vi "TLB Native Dynamic Events ver 0.13d.vi"() -> ()   [LabVIEW 2018]
uses:
  Labview Training Phase 2/Enum Controls/States for Action Engine.ctl
  TLB Type Definitions/State Type Definitions, for 0.26d versions and later.ctl
  TLB Type Definitions/Intruction Type Definitions.ctl
  TLB Type Definitions/Encoder cluster.ctl
  TLB Type Definitions/PING CLUSTER.ctl
  <vilib>/Studica/Studica Toolkit/NavX/NavX.lvlib
  <vilib>/Studica/Studica Toolkit/Background/DIO Channel.ctl
  Underlying VI's/NavX VI/navX type def.ctl
  <vilib>/myRIO/Instrument Drivers/Utilities/Utilities.lvlib
  <vilib>/Studica/Studica Toolkit/Background/I2C Channel.ctl
  TLB Type Definitions/Vision cluster.ctl
  <vilib>/NI_Real-Time Target Support.lvlib
  TLB Type Definitions/Stepper cluster.ctl
  Experimental VI's/Archived VI's/MOTOR CONTROL NO PID Type Def.ctl
  Underlying VI's/I2C Master VI/I2C MASTER Type Def.ctl
  Underlying VI's/I2C Master VI/I2C_MASTER_WRITE_NEW Type Def.ctl
  Underlying VI's/Webcam FGV Low level ver/State control.ctl
  <vilib>/userdefined/High Color/IMAQdx.ctl
  Underlying VI's/I2C Master VI/Arduino_Interfacing.ctl
  TLB Type Definitions/Yaw Cluster.ctl
  Experimental VI's/Archived VI's/MOTOR CONTROL NO PID AE DATA ENTRY MODE Type def.ctl
  Experimental VI's/Archived VI's/MOTOR CONTROL NO PID AE DIRECTIONS type def.ctl
  <vilib>/Utility/RT CPU Load.ctl
panel:
  out "Task selection":u8
  out "Object Center Coordinates":cluster{"x":sgl, "y":sgl}
  out "Object detection cluster":T1
  in  "Object recognition mode":enum16{"Ball", "Soap", "Gel", "Pipe", "None"}(ring)
  out "NavX Readings":T2
  out "Arduino Data":T3
  out "CPU loads":T4[](array[typedef]) {"ISR (%)" format="%#.2f"; "Idle (%)" format="%#.2f"; "Background (%)" format="%#.2f"; "Normal (%)" format="%#.2f"; "Above Normal (%)" format="%#.2f"; "High (%)" format="%#.2g"; "Timed Structures (%)" format="%#.2g"; "Time Critical (%)" format="%#.2g"; "Total (%)" format="%#.2g"}
  in  "Red LED":bool
  out "Detect?":bool
  out "TASK ENABLE":bool
  out "Rising Edge":bool
  in  "Green LED":bool
  out "Object detected?":bool
  out "I2C Error":errorcluster
  out "State Logic":T5=enum."Startup"
  out "elements":T6[](array[typedef])
  in  "STOP TASK":bool
  in  "OK Button":bool
  in  "STOP":bool
  out "error out":errorcluster
  out "Action Queue Items":i32
  out "State Logic Queue Items":i32
  out "Action Queues items":string[](array[string])=["Hardware reset", "Software reset", ""]
  out "Action State":string
  # "TLB FRAMEWORK STATUS"
  # "System Health Status Update"
  # "Test Programme written by Calvin Loke    Dated: 28 Aug 2019\nTest Programme revised by Dr Alex See   Dated 30 Aug 2019\n\nProgramme version:   TLB Native Dynamic Events ver 0.04b.vi"
  # "VISION"
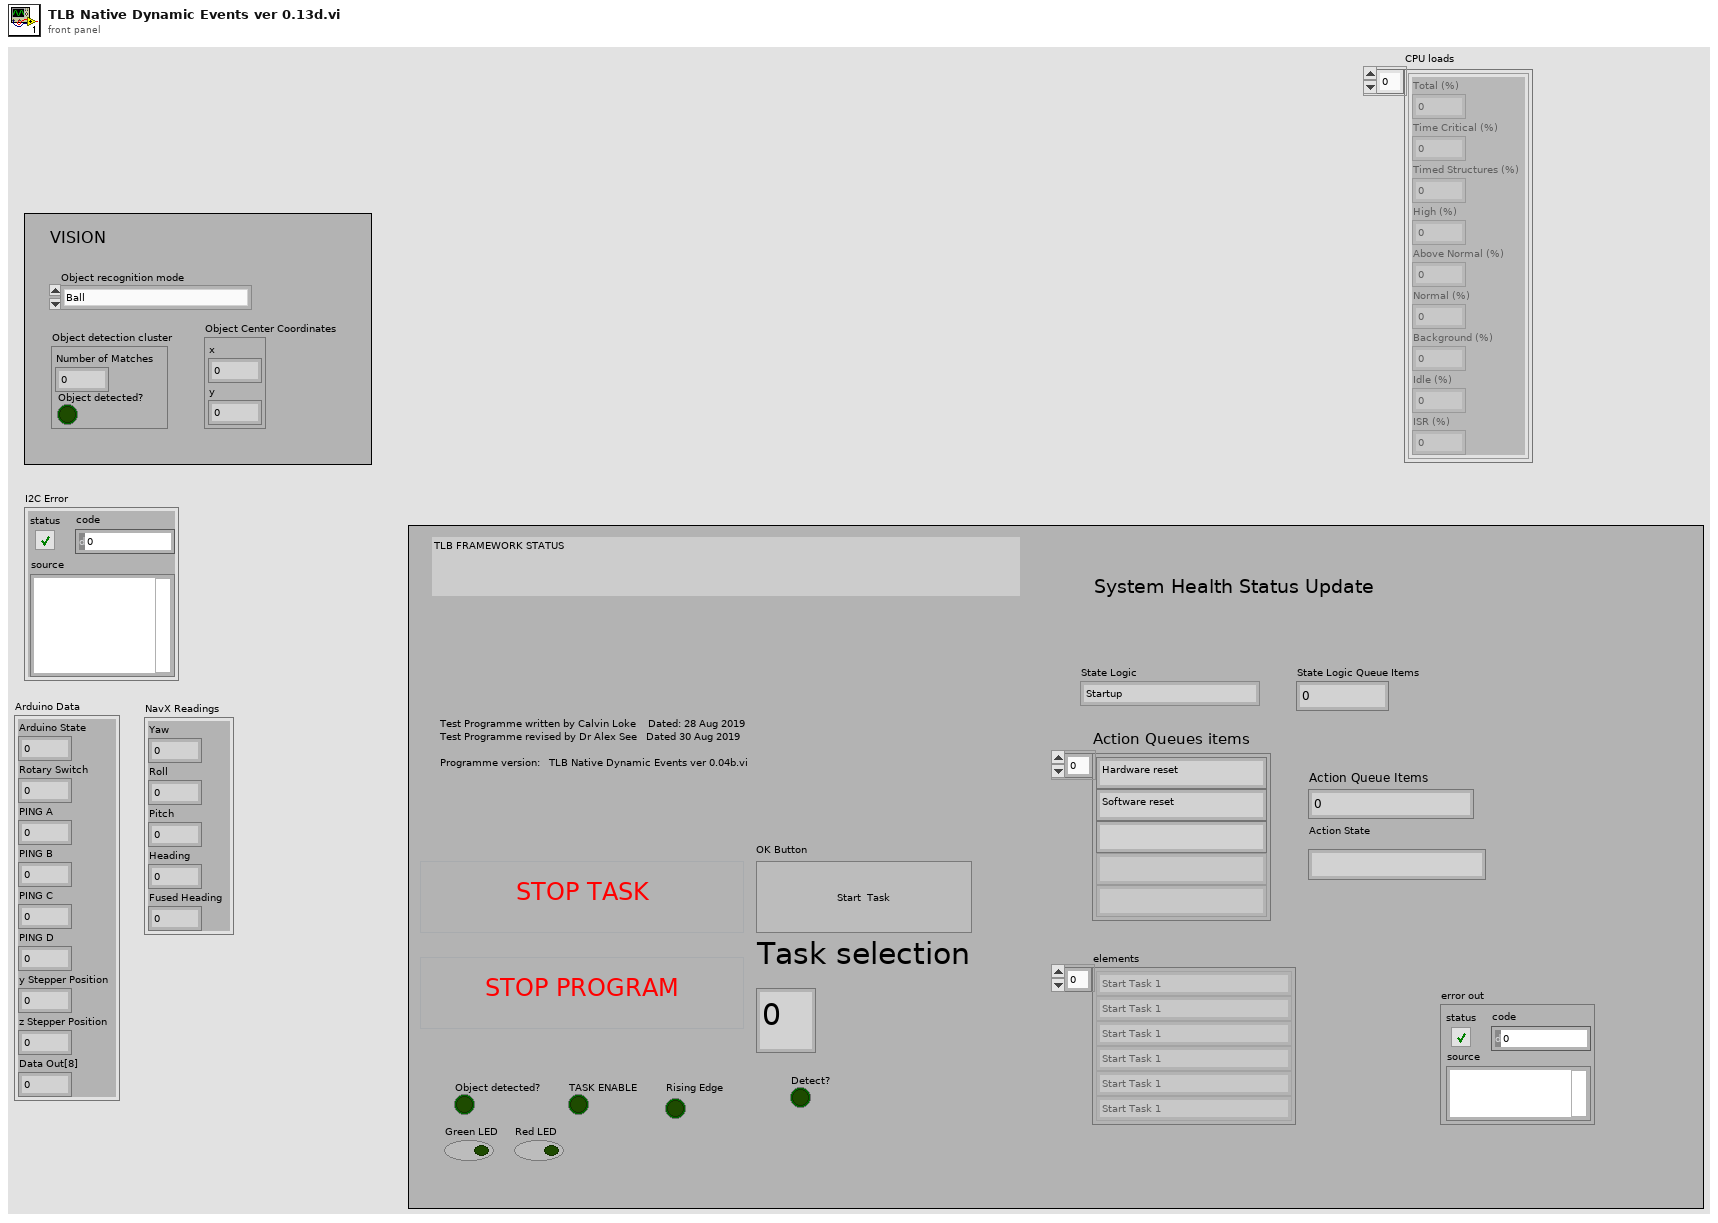
[diagram p1: front panel]
types:
  T1 = cluster{"Number of Matches":i32, "Object detected?":bool}
  T2 = cluster{"Yaw":dbl, "Roll":dbl, "Pitch":dbl, "Heading":dbl, "Fused Heading":dbl}
  T3 = cluster{"Arduino State":u8, "Rotary Switch":u8, "PING A":u8, "PING B":u8, "PING C":u8, "PING D":u8, "y Stepper Position":u8, "z Stepper Position":u8, "Data Out[8]":u8}
  T4 = typedef "NI_Real-Time Target Support.lvlib/RT CPU Load.ctl" = cluster{"Total (%)":dbl, "Time Critical (%)":dbl, "Timed Structures (%)":dbl, "High (%)":dbl, "Above Normal (%)":dbl, "Normal (%)":dbl, "Background (%)":dbl, "Idle (%)":dbl, "ISR (%)":dbl}
  T5 = typedef "State Type Definitions.ctl" = enum16{"None", "Startup", "Move to Angle", "True Stop", "Idle", "Shutdown", "Task 1A", "Task 1B", "Task 2:Raise Arm", "Task 2:Sensor Mode", "Task 2:Reverse Mode", "Task 3", "Task 4_A", "Task 4_B", "Task 4_C", "Task 4_D", "Task 5A", "Task 5B", "Task 5C", "Task 5D", "Task 5E: POSITION ARM", "Task 5F: ARM GRAB HEIGHT", "Task 5G: CLOSE CLAW", "Task 5H: RAISE ARM", "Task 6_A", "Task 6_B", "Task 7", "Task 8A: RAISE ARM", "Task 8B: MOVE TO BOX", "Task 8C: CAM BURST", "Task 8D: PROCESS IMAGE", "Task 8E: ROBOT ADJUST", "Task 8F: CAM BURST 2", "Task 8G: PROCESS IMAGE 2", "Task 8H: ARM ADJUST", "Task 8I: ARM GRAB HEIGHT", "Task 8J: CLOSE CLAW", "Task 8K: RAISE MY SWORD", "Task 9A: Raise Arm", "Task 9B: Rotate to Angle", "Task 9C: Detect Box", "Task 9D: MOVE FORWARD", "Task 9E: MOVE LEFT", "Task 9F: SCAN IMAGE", "Task 9G: PROCESS COLOUR", "Task 9H: MOVE RIGHT", "Task 9I: SCAN IMAGE", "Task 9J: PROCESS COLOUR", "Task 9K: ROTATE 90 CW", "Task 9L: MOVE FORWARD", "Task 9M: MOVE RIGHT", "Task 9N: SCAN IMAGE", "Task 9O: PROCESS COLOUR", "Task 9P: MOVE RIGHT", "Task 9Q: SCAN IMAGE", "Task 9R: PROCESS COLOUR", "Task A1: Raise Arm", "Task A2: Rotate to Angle", "Task A3: Move Forward", "Task A4: Rotate CW 90"}
  T6 = typedef "Intruction Type Definitions.ctl" = enum16{"None", "Start Task 1", "Start Task 2", "Start Task 3", "Start Task 4", "Start Task 5", "Start Task 6", "Start Task 7", "Start Task 8 - BALL", "Start Task 8 - Gel", "Start Task 8 - Pipe", "Start Task 8 - Soap", "Start Task 9", "Start Task A", "Start Task B", "Exit"}
  T7 = typedef "Yaw Cluster.ctl" = cluster{"Yaw":dbl, "Compass":dbl}
  T8 = typedef "Stepper cluster.ctl" = cluster{"y Stepper Position":u8, "z Stepper Position":u8}
  T9 = typedef "DIO Channel.ctl" = enum16{"Not Connected", "A/DIO1", "A/DIO2", "A/DIO3", "A/DIO4", "A/DIO5", "A/DIO6", "A/DIO7", "A/DIO13", "B/DIO1", "B/DIO2", "B/DIO3", "B/DIO4", "B/DIO5", "B/DIO6", "B/DIO7", "B/DIO13", "C/DIO0", "C/DIO1", "C/DIO2", "C/DIO3", "C/DIO4", "C/DIO5", "C/DIO6", "C/DIO7"}
  T10 = typedef "Vision cluster.ctl" = cluster{"Recognized Object":bool, "Object X coordinate":dbl, "Object Y coordinate":dbl}
  T11 = typedef "PING CLUSTER.ctl" = cluster{"PING_A":u8, "PING_B":u8, "PING_C":u8, "PING_D":u8}
  T12 = typedef "Encoder cluster.ctl" = cluster{"xDistance":dbl, "yDistance":dbl, "wDistance":dbl}
  T13 = cluster{"DIO Channel":T9, "FPGA VI Reference Out":refnum<k20>}
  T14 = typedef "navX type def.ctl" = enum16{"Get i2C reference", "Read Values", "Zero Yaw"}
  T15 = typedef "Arduino_Interfacing.ctl" = enum16{"Initialize", "Write to Arduino", "Read From Arduino"}
  T16 = typedef "I2C Channel.ctl" = enum16{"Not Connected", "A", "B"}
  T17 = typedef "States for Action Engine.ctl" = enum16{"Initialize", "Write", "Read"}
  T18 = cluster{"I2C Ref Out":cluster{"I2C Channel":T16, "FPGA VI Reference Out":refnum<k20>}, "Connected":bool, "Slave Address (7-bit)":u8, "Registry":u8[]}
  T19 = typedef "IMAQ Image.ctl" = refnum<image>
  T20 = typedef "State Type Definitions.ctl" = enum16{"None", "Startup", "Move to Angle", "True Stop", "Idle", "Shutdown", "Task 1", "Task 2:Raise Arm", "Task 2:Sensor Mode", "Task 2:Reverse Mode", "Task 3", "Task 4_A", "Task 4_B", "Task 4_C", "Task 4_D", "Task 5A: ARM CAM HEIGHT", "Task 5B: MOVE TO BOX", "Task 5C: CAM BURST", "Task 5D: PROCESS IMAGE", "Task 5E: POSITION ARM", "Task 5F: ARM GRAB HEIGHT", "Task 5G: CLOSE CLAW", "Task 5H: RAISE ARM", "Task 6_A", "Task 6_B", "Task 7", "Task 8A: RAISE ARM", "Task 8B: MOVE TO BOX", "Task 8C: CAM BURST", "Task 8D: PROCESS IMAGE", "Task 8E: ROBOT ADJUST", "Task 8F: CAM BURST 2", "Task 8G: PROCESS IMAGE 2", "Task 8H: ARM ADJUST", "Task 8I: ARM GRAB HEIGHT", "Task 8J: CLOSE CLAW", "Task 8K: RAISE MY SWORD", "Task 9A: Raise Arm", "Task 9B: Rotate to Angle", "Task 9C: Detect Box", "Task 9D: MOVE FORWARD", "Task 9E: MOVE LEFT", "Task 9F: SCAN IMAGE", "Task 9G: PROCESS COLOUR", "Task 9H: MOVE RIGHT", "Task 9I: SCAN IMAGE", "Task 9J: PROCESS COLOUR", "Task 9K: ROTATE 90 CW", "Task 9L: MOVE FORWARD", "Task 9M: MOVE RIGHT", "Task 9N: SCAN IMAGE", "Task 9O: PROCESS COLOUR", "Task 9P: MOVE RIGHT", "Task 9Q: SCAN IMAGE", "Task 9R: PROCESS COLOUR"}
  T21 = typedef "State Type Definitions.ctl" = enum16{"None", "Startup", "Move to Angle", "True Stop", "Idle", "Shutdown", "Task 1", "Task 2", "Task 3", "Task 4_A", "Task 4_B", "Task 4_C", "Task 5", "Task 6_A", "Task 6_B", "Task 7", "Task 8", "Task 9", "Task A", "Task B"}
  T22 = typedef "MOTOR CONTROL NO PID AE DIRECTIONS type def.ctl" = enum16{"y-axis movement", "x-axis movement", "Rotate", "Stop"}
  T23 = typedef "MOTOR CONTROL NO PID AE DATA ENTRY MODE Type def.ctl" = enum16{"Initialize", "Reset Encoders", "Write to motors", "Read from Encoders"}
  T24 = typedef "I2C_MASTER_WRITE_NEW Type Def.ctl" = enum16{"Ultrasonic sensors", "Stepper origin", "zStepper 13.3k", "zStepper 13k", "zStepper 12k", "zStepper 11k", "zStepper 10k", "zStepper 9k", "zStepper 8k", "zStepper 7k", "zStepper 6k", "zStepper 5k", "zStepper 4k", "zStepper 3k", "zStepper 2k", "zStepper 1k", "zStepper 900", "zStepper 800", "zStepper 700", "zStepper 600", "zStepper 500", "zStepper 400", "zStepper 300", "zStepper 200", "zStepper 100", "zStepper 0", "yStepper control", "Open Claw", "Close Claw", "Soft Reset"}
  T25 = typedef "State control.ctl" = enum16{"Initialise", "Start camera", "Continuous Acquisition ", "Stop camera", "Dispose all"}
  T26 = typedef "IMAQdx.ctl" = refnum<k21>
  T27 = cluster{"xSpeed":dbl, "ySpeed":dbl, "wSpeed":dbl, "xDistance":dbl, "yDistance":dbl, "wDistance":dbl}
  T28 = typedef "MOTOR CONTROL NO PID Type Def.ctl" = enum16{"Init", "Front Back", "Left Right", "Rotate", "Stop", "Latch"}
  T29 = typedef "I2C MASTER Type Def.ctl" = enum16{"Last State", "Mode 0", "Mode 1", "Mode 2", "Mode 3", "Mode 4", "Mode 5", "Mode 6", "Mode 7", "Mode 8", "Mode 9", "Mode 10"}
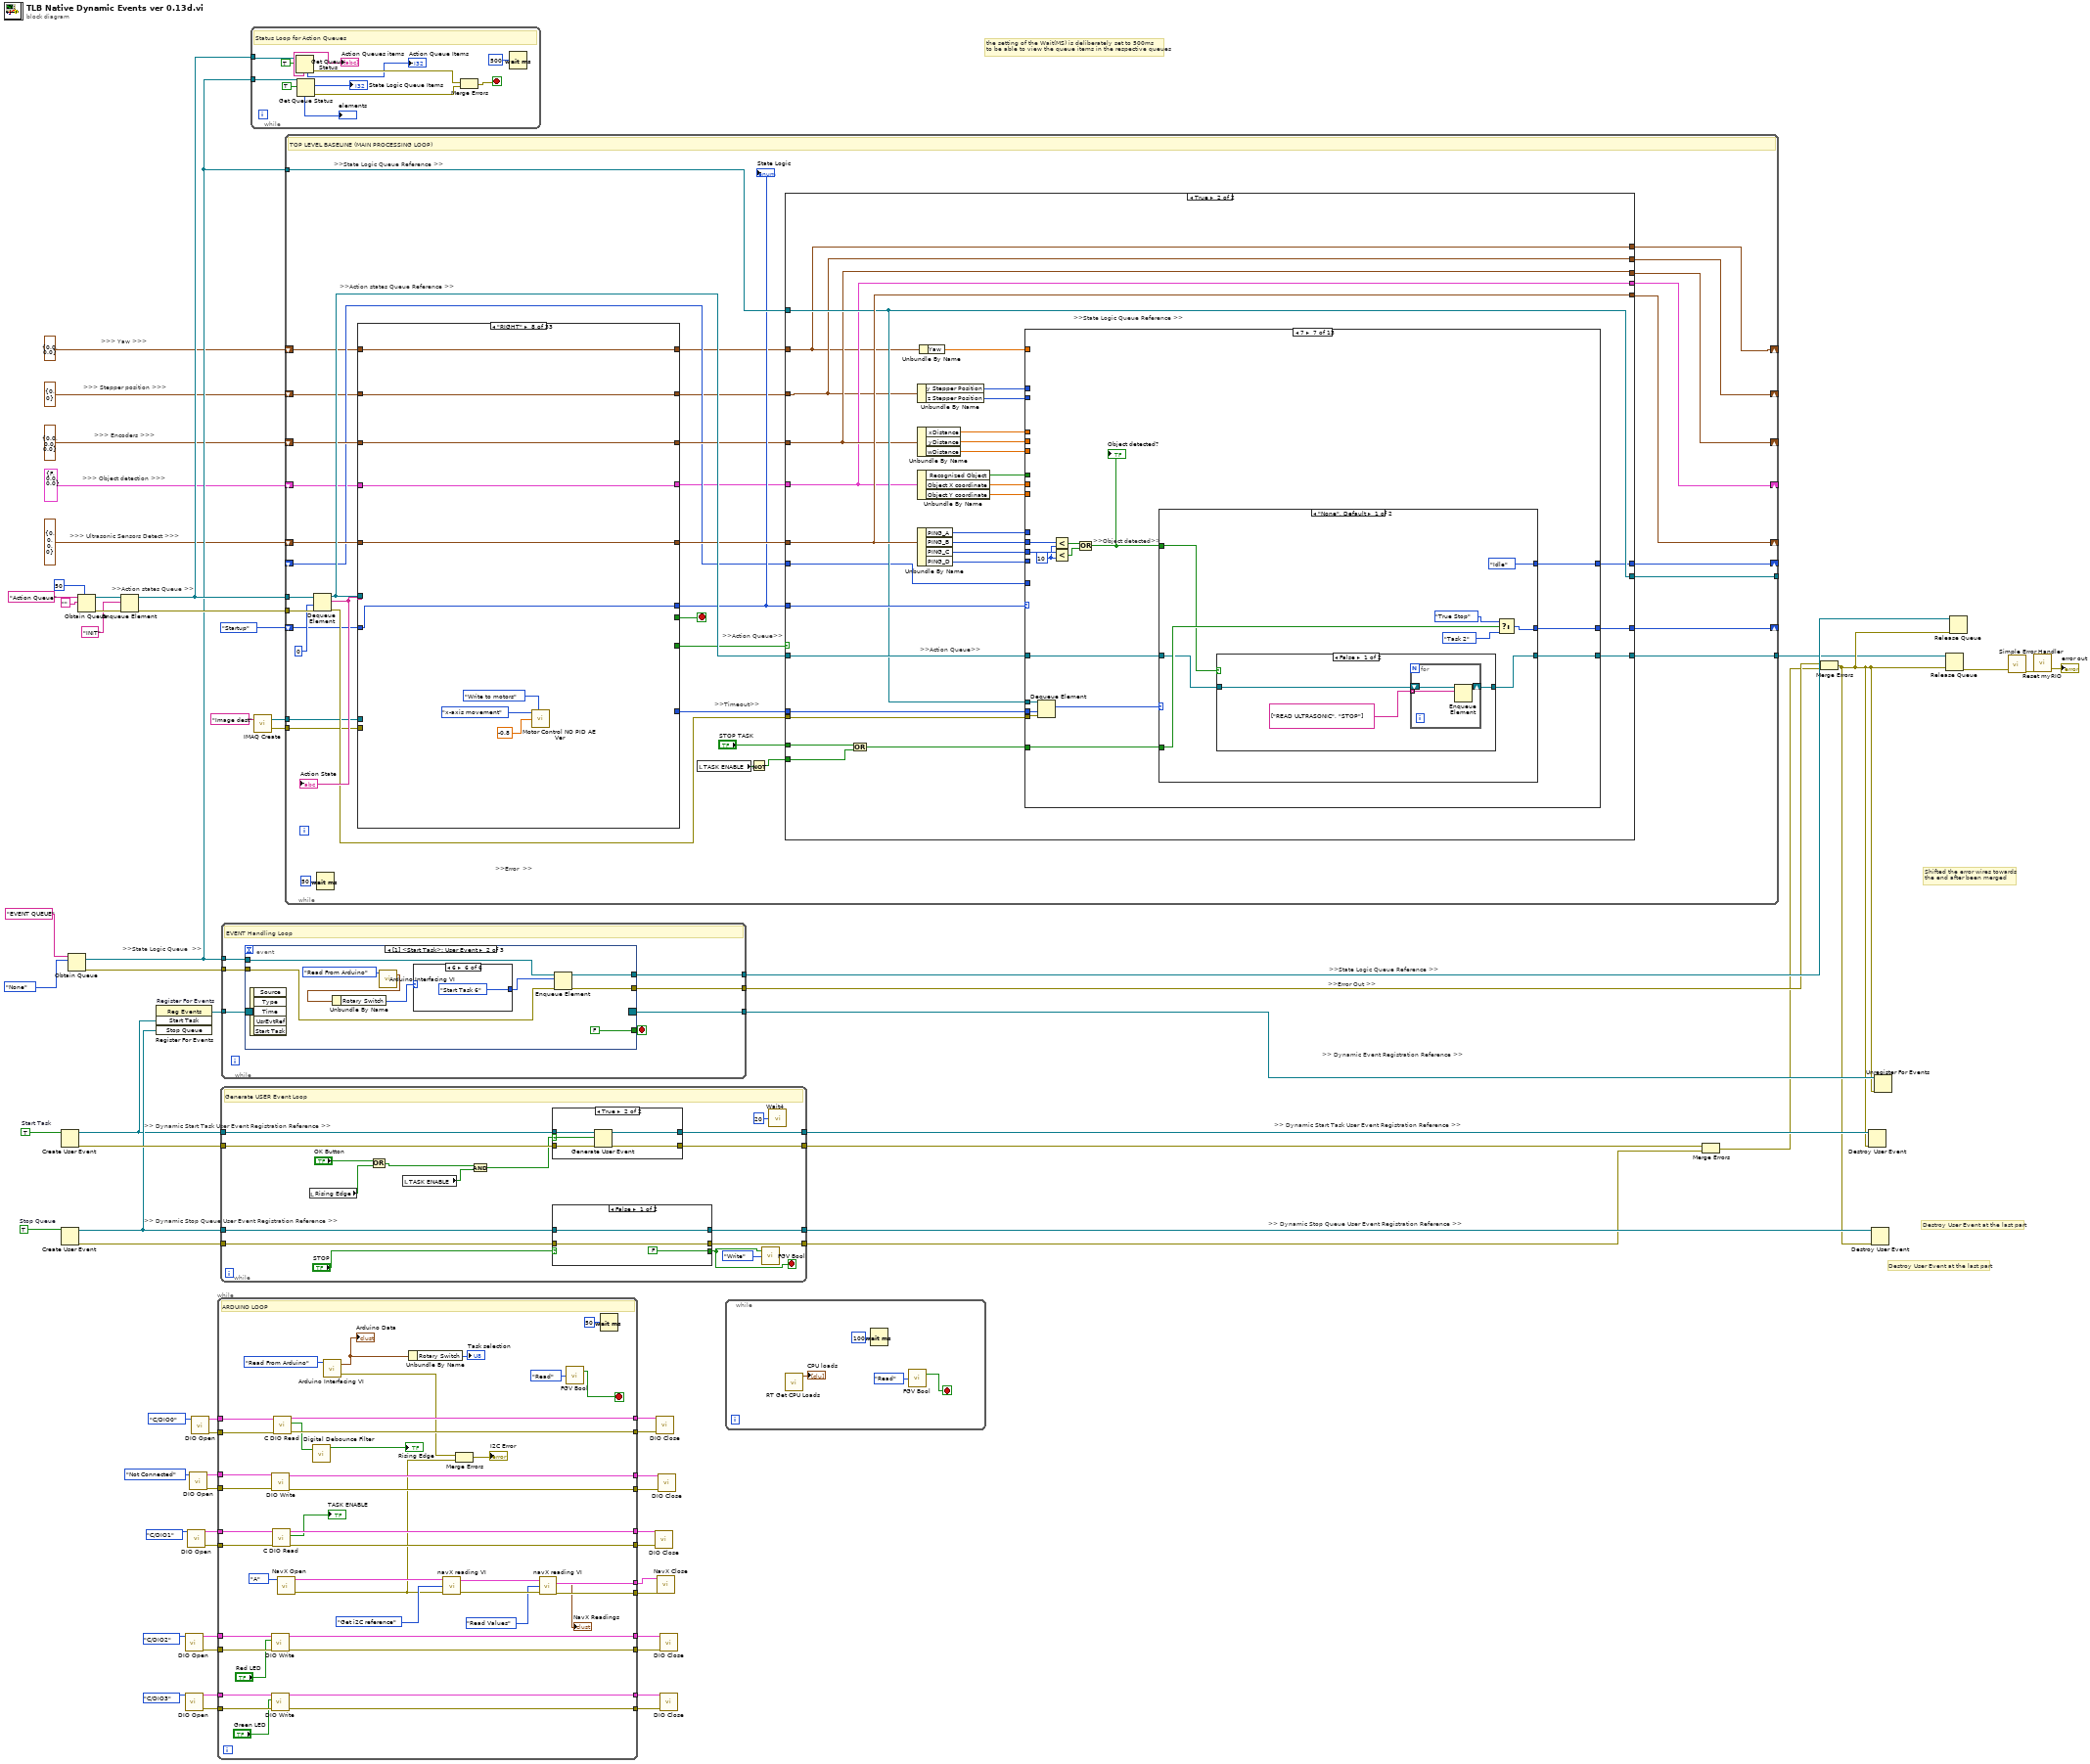
[diagram p0: block diagram]
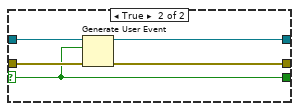
[diagram p2: hidden frame]
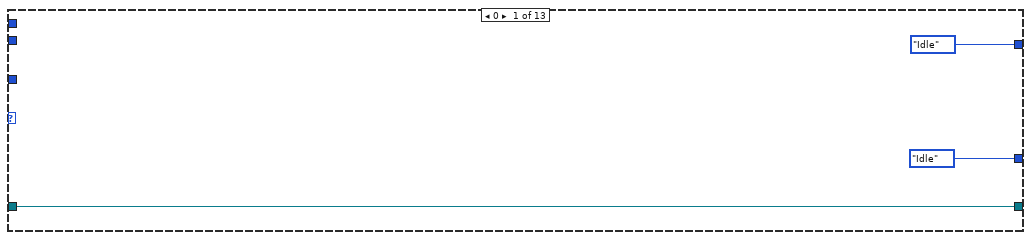
[diagram p5: hidden frame]
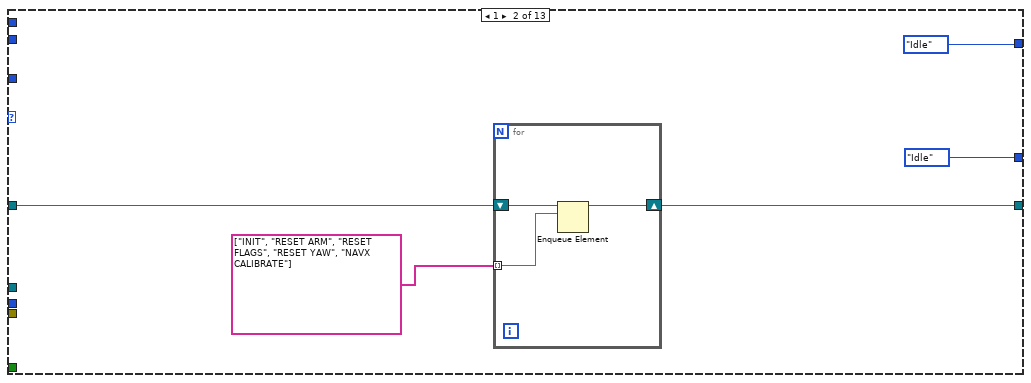
[diagram p6: hidden frame]
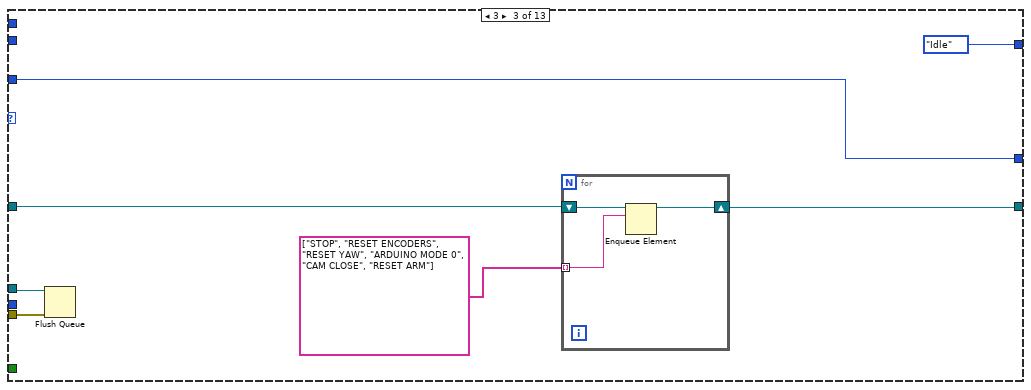
[diagram p7: hidden frame]
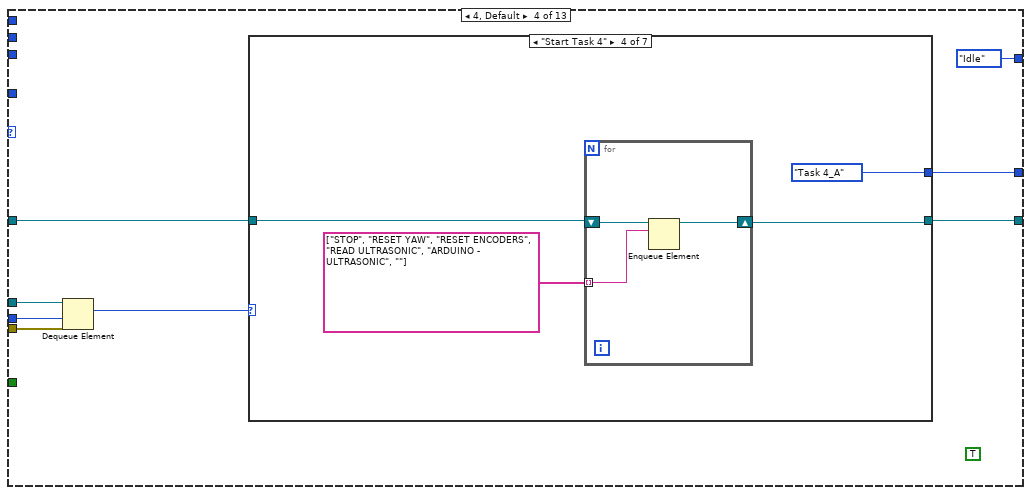
[diagram p8: hidden frame]
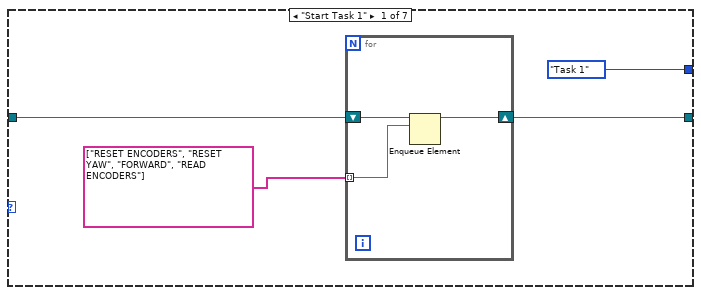
[diagram p9: hidden frame]
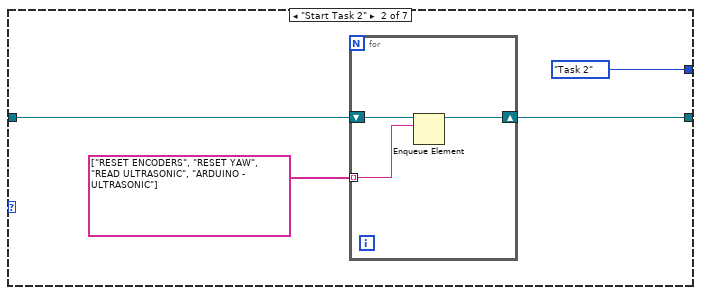
[diagram p10: hidden frame]
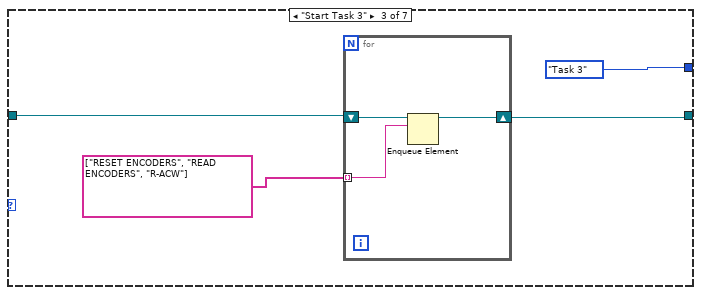
[diagram p11: hidden frame]
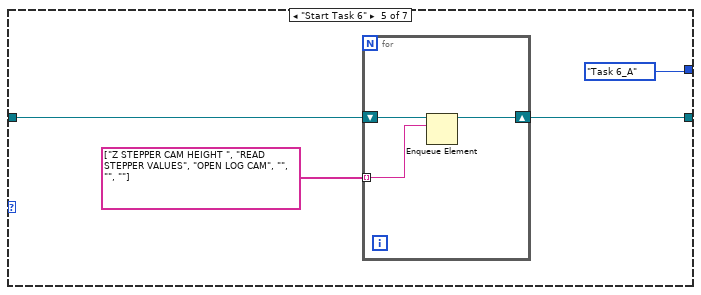
[diagram p12: hidden frame]
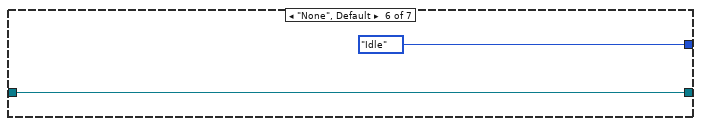
[diagram p13: hidden frame]
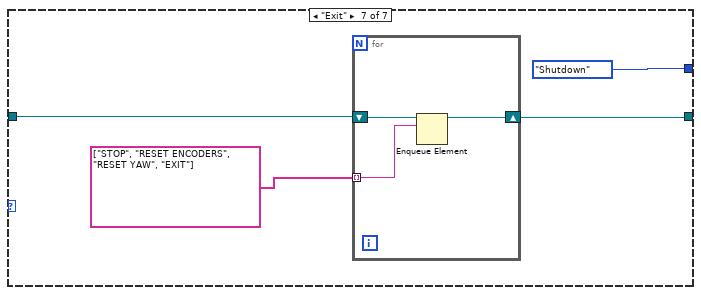
[diagram p14: hidden frame]
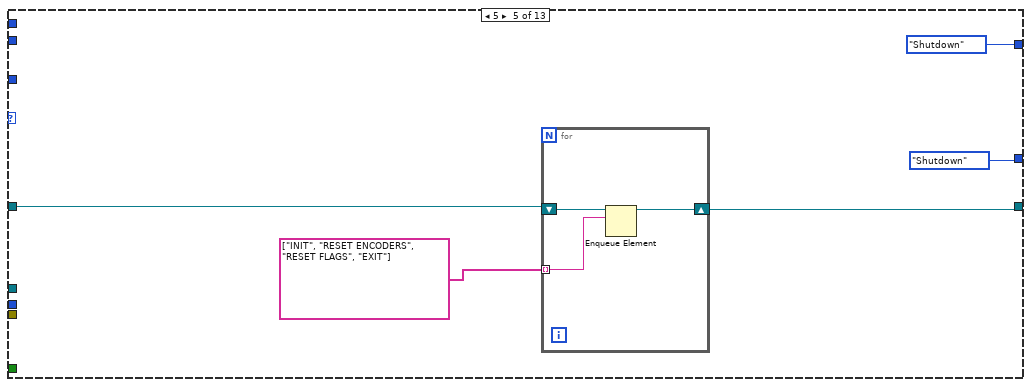
[diagram p15: hidden frame]
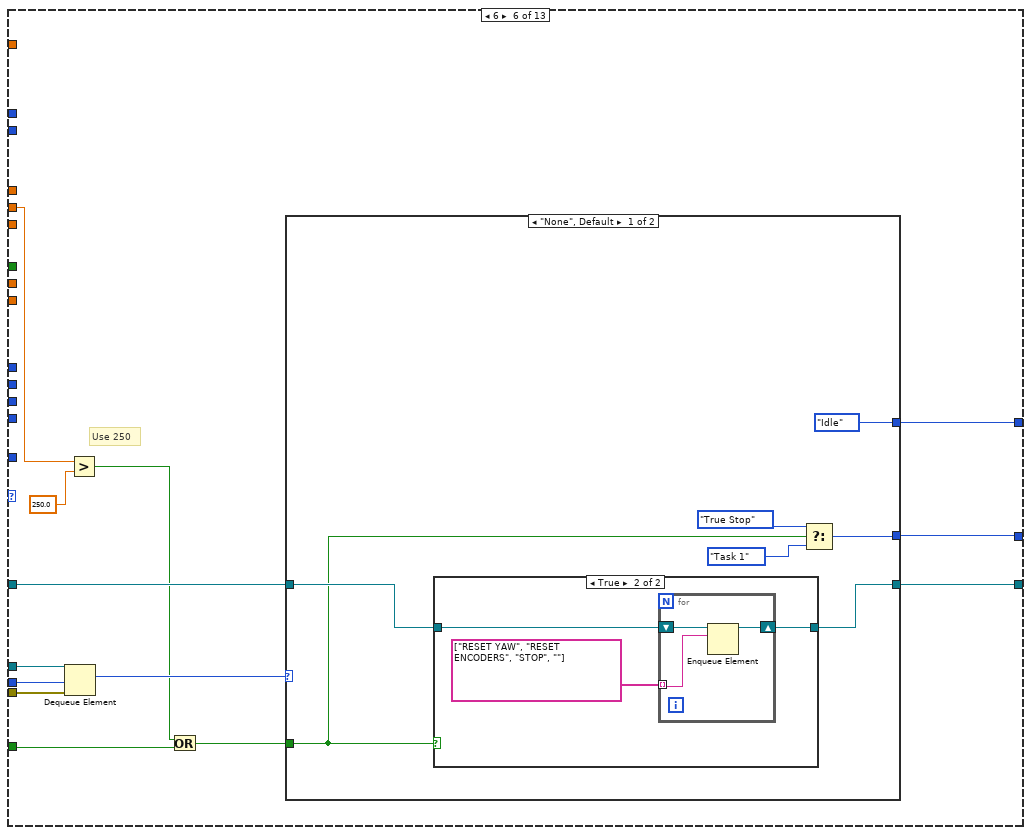
[diagram p16: hidden frame]
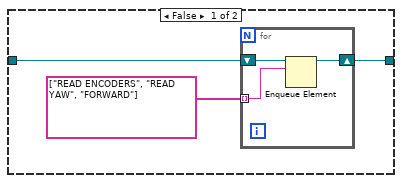
[diagram p17: hidden frame]
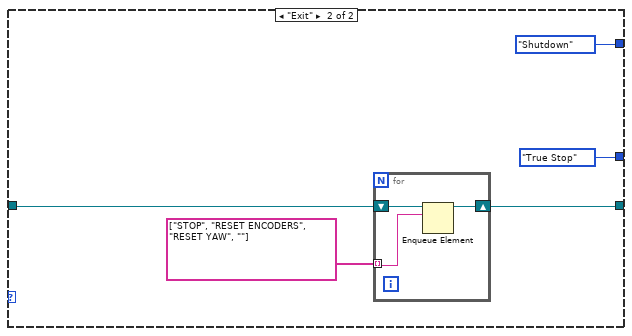
[diagram p18: hidden frame]
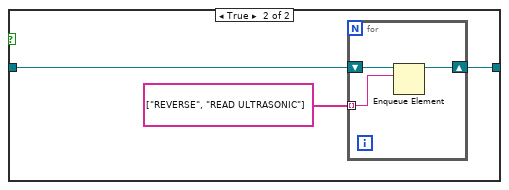
[diagram p19: hidden frame]
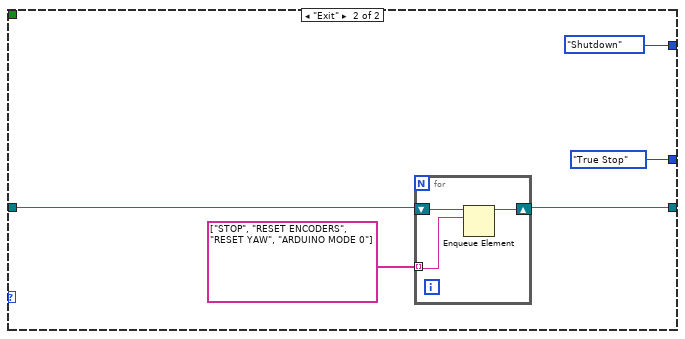
[diagram p20: hidden frame]
diagram:
  w68 = TRUE  # Stop Queue
  w67 = TRUE  # Start Task
  # ">>> Yaw >>>"
  # ">>> Stepper position >>>"
  # ">>> Encoders >>>"
  # ">>> Object detection >>>"
  # ">>> Ultrasonic Sensors Detect >>>"
  # "the setting of the Wait(MS) is deliberately set to 500ms\nto be able to view the queue items in the respective queues"
  # ">>Error Out >>"
  # ">> Dynamic Stop Queue User Event Registration Reference >>"
  # ">> Dynamic Start Task User Event Registration Reference >>"
  # ">> Dynamic Stop Queue User Event Registration Reference >>"
  # ">> Dynamic Start Task User Event Registration Reference >>"
  # ">> Dynamic Event Registration Reference >>"
  # ">>Action states Queue >>"
  # ">>State Logic Queue  >>"
  # ">>State Logic Queue Reference >>"
  # "Destroy User Event at the last part"
  # "Destroy User Event at the last part"
  # "Shifted the error wires towards\nthe end after been merged"
  n1 = Create User Event(user event datatype=w67) -> (user event=w59:refnum<user-event>, error out=w64:errorcluster)  [unwired: 1 in]
  n2 = Create User Event(user event datatype=w68) -> (user event=w60:refnum<user-event>, error out=w63:errorcluster)  [unwired: 1 in]
  n3 = Obtain Queue(name (unnamed)="EVENT QUEUE", element data type=Intruction_Type_Definitions."None" ("Enum")) -> (queue out=w45:refnum<queue>, error out=w51:errorcluster)  [unwired: 3 in, 1 out]
  n4 = Obtain Queue(max queue size (-1, unlimited)=50, name (unnamed)="Action Queue", element data type="") -> (queue out=w54:refnum<queue>, error out=w50:errorcluster)  [unwired: 2 in, 1 out]
  n5 = Enqueue Element(queue=w54, element="INIT", error in (no error)=w50) -> (queue out=w46:refnum<queue>, error out=w49:errorcluster)  [unwired: 1 in, 1 out]
  n6 = register-events "Register For Events"(w59, w60) -> (reference out=w58:refnum<event-registration>)  [unwired: 2 in, 1 out]
  n7 = call <vilib>:"DIO Open.vi"("DIO Channel"=DIO_Channel."C/DIO2") -> ("error out"=w12:errorcluster, "DIO Info Out"=w13:T13)  [unwired: 9 in]
  n8 = call <vilib>:"DIO Open.vi"("DIO Channel"=DIO_Channel."C/DIO3") -> ("error out"=w7:errorcluster, "DIO Info Out"=w8:T13)  [unwired: 9 in]
  n9 = call <vilib>:"DIO Open.vi"("DIO Channel"=DIO_Channel."C/DIO1") -> ("error out"=w23:errorcluster, "DIO Info Out"=w24:T13)  [unwired: 9 in]
  n10 = call <vilib>:"DIO Open.vi"("DIO Channel"=DIO_Channel."Not Connected") -> ("error out"=w28:errorcluster, "DIO Info Out"=w30:T13)  [unwired: 9 in]
  n11 = call <vilib>:"DIO Open.vi"("DIO Channel"=DIO_Channel."C/DIO0") -> ("error out"=w33:errorcluster, "DIO Info Out"=w36:T13)  [unwired: 9 in]
  n12 = while {
    tunnel: w36 -> [w108]
    tunnel: [w107] -> w34
    tunnel: w33 -> [w106]
    tunnel: [w105] -> w32
    tunnel: w30 -> [w101]
    tunnel: [w100] -> w29
    tunnel: w28 -> [w99]
    tunnel: [w98] -> w27
    tunnel: [w97] -> w25
    tunnel: w24 -> [w96]
    tunnel: w23 -> [w95]
    tunnel: [w94] -> w22
    tunnel: w13 -> [w88]
    tunnel: w12 -> [w87]
    tunnel: [w86] -> w11
    tunnel: [w85] -> w10
    tunnel: w8 -> [w83]
    tunnel: w7 -> [w82]
    tunnel: [w81] -> w6
    tunnel: [w80] -> w5
    tunnel: [w74] -> w2
    tunnel: [w73] -> w3
    stop <- w110 stop-if-true
    # "ARDUINO LOOP"
    n13 = call <vilib>:"DIO Write.vi"("error in (no error)"=w87, "Input"="Red LED", "DIO Info In"=w88) -> ("error out"=w85:errorcluster, "DIO Info Out"=w86:T13)  [unwired: 7 in]
    n14 = call <vilib>:"DIO Write.vi"("error in (no error)"=w82, "Input"="Green LED", "DIO Info In"=w83) -> ("error out"=w80:errorcluster, "DIO Info Out"=w81:T13)  [unwired: 7 in]
    n15 = call <vilib>:"DIO Write.vi"("error in (no error)"=w99, "DIO Info In"=w101) -> ("error out"=w98:errorcluster, "DIO Info Out"=w100:T13)  [unwired: 8 in]
    n16 = call <vilib>:"C DIO Read.vi"("error in (no error)"=w95, "DIO Info In in"=w96) -> ("error out"=w94:errorcluster, "IN"=→"TASK ENABLE":bool, "DIO Info In out"=w97:T13)  [unwired: 7 in]
    n17 = call <vilib>:"C DIO Read.vi"("error in (no error)"=w106, "DIO Info In in"=w108) -> ("error out"=w105:errorcluster, "IN"=w103:bool, "DIO Info In out"=w107:T13)  [unwired: 7 in]
    n18 = call <vilib>:"NavX Open.vi"("I2C Channel"=I2C_Channel."A") -> ("error out"=w90:errorcluster, "NavX Info"=w92:T18)  [unwired: 9 in]
    n19 = call "Digital Debounce Filter.vi"("Boolean input"=w103) -> ("Rising Edge"=→"Rising Edge":bool)  [unwired: 1 in, 2 out]
    n20 = call "Arduino Interfacing VI.vi"("AE Mode"=Arduino_Interfacing."Read From Arduino") -> ("error out"=w77:errorcluster, "Arduino Data"=w70:T3)  [unwired: 3 in]
    "Arduino Data" <- w70
    n21 = Unbundle By Name(w70) -> ("Rotary Switch"=→"Task selection":u8)
    n22 = call "navX reading VI.vi"("NavX Info In"=w92, "Mode"=navX_type_def."Get i2C reference", "error in (no error)"=w90) -> ("NavX Info Out"=w76:T18, "Error Out"=w75:errorcluster)  [unwired: 2 out]
    n23 = Merge Errors(w77, w90) -> (→"I2C Error":errorcluster)
    n24 = call "navX reading VI.vi"("NavX Info In"=w76, "Mode"=navX_type_def."Read Values", "error in (no error)"=w75) -> ("NavX Info Out"=w74:T18, "NavX Readings"=→"NavX Readings":T2, "Error Out"=w73:errorcluster)  [unwired: 1 out]
    n25 = call "FGV Bool.vi"("Init/Read/Write State"=States_for_Action_Engine."Read") -> ("Output node"=w110:bool)  [unwired: 2 in, 1 out]
    n26 = Wait (ms)(milliseconds to wait=u32 50) -> ()  [unwired: 1 out]
  }
  n27 = while {
    tunnel: w59 -> [w128]
    tunnel: w60 -> [w127]
    tunnel: [w126] -> w66
    tunnel: [w125] -> w65
    tunnel: w64 -> [w124]
    tunnel: [w123] -> w62
    tunnel: w63 -> [w122]
    tunnel: [w121] -> w61
    stop <- w119 stop-if-true
    # "Generate USER Event Loop"
    n28 = local read "Rising Edge"() -> (w115:bool)
    n29 = Or(x="OK Button", y=w115) -> (x .or. y?=w114:bool)
    n30 = local read "TASK ENABLE"() -> (w113:bool)
    n31 = And(x=w114, y=w113) -> (x .and. y?=w112:bool)
    n32 = case shown="True" w112 {
      selector: w112 -> [_ w139]
      tunnel: w128 -> [w138 w143]
      tunnel: [w138 w142] -> w125
      tunnel: w124 -> [w137 w141]
      tunnel: [w137 w140] -> w123
      frame False {
      }
      frame True {
        n33 = Generate User Event(user event=w143, event data cluster=w139, error in=w141) -> (user event out=w142:refnum<user-event>, error out=w140:errorcluster)  [unwired: 1 in]
      }
    }
    n34 = case shown="False" "STOP" {
      selector: "STOP" -> [_ w132]
      tunnel: w127 -> [w131 w136]
      tunnel: [w131 w135] -> w126
      tunnel: w122 -> [w130 w134]
      tunnel: [w130 w133] -> w121
      tunnel: [FALSE w132] -> w119
      frame False {
      }
      frame True {
        n35 = Generate User Event(user event=w136, event data cluster=w132, error in=w134) -> (user event out=w135:refnum<user-event>, error out=w133:errorcluster)  [unwired: 1 in]
      }
    }
    n36 = call "FGV Bool.vi"("Init/Read/Write State"=States_for_Action_Engine."Write", "Input Node"=w119) -> ()  [unwired: 1 in, 2 out]
    n37 = call "Wait4"("Count(uSec)"=u32 20) -> ()  [unwired: 1 out]
  }
  n38 = while {
    tunnel: w58 -> [w150]
    tunnel: [w149] -> w57
    tunnel: w45 -> [w147]
    tunnel: [w146] -> w56
    tunnel: w51 -> [w145]
    tunnel: [w144] -> w48
    stop <- w148 stop-if-true
    # "EVENT Handling Loop"
    n39 = event shown="[1] <Start Task>: User Event" {
      selector: w150 -> [_ _ _]
      dyn-events: [_ _ _] -> w149
      timeout: _ -> [_ _ _]
      tunnel: [FALSE FALSE w177] -> w148
      tunnel: w147 -> [w155 w164 w175]
      tunnel: [w154 w163 w176] -> w146
      tunnel: w145 -> [w153 w162 w174]
      tunnel: [w152 w161 w173] -> w144
      event Timeout {
        n40 = event-data() -> ()  [unwired: 1 in, 3 out]
        n41 = Enqueue Element(queue=w155, element=Intruction_Type_Definitions."None" ("Enum"), error in (no error)=w153) -> (queue out=w154:refnum<queue>, error out=w152:errorcluster)  [unwired: 1 in, 1 out]
      }
      event User Event {
        n42 = event-data() -> ()  [unwired: 1 in, 5 out]
        n43 = call "Arduino Interfacing VI.vi"("AE Mode"=Arduino_Interfacing."Read From Arduino") -> ("Arduino Data"=w158:T3)  [unwired: 3 in, 1 out]
        n44 = Unbundle By Name(w158) -> ("Rotary Switch"=w157:u8)
        n45 = case shown="6" w157 {
          tunnel: [Intruction_Type_Definitions."None" ("Enum") Intruction_Type_Definitions."Start Task 1" ("Enum") Intruction_Type_Definitions."Start Task 2" ("Enum") Intruction_Type_Definitions."Start Task 3" ("Enum") Intruction_Type_Definitions."Start Task 4" ("Enum") Intruction_Type_Definitions."Start Task 6" ("Enum")] -> w160
          frame 0, Default {
          }
          frame 1 {
          }
          frame 2 {
          }
          frame 3 {
          }
          frame 4 {
          }
          frame 6 {
          }
        }
        n46 = Enqueue Element(queue=w164, element=w160, error in (no error)=w162) -> (queue out=w163:refnum<queue>, error out=w161:errorcluster)  [unwired: 1 in, 1 out]
      }
      event User Event {
        n47 = event-data() -> ("Stop Queue"=w177:bool)  [unwired: 1 in, 4 out]
        n48 = Enqueue Element At Opposite End(queue=w175, element=Intruction_Type_Definitions."Exit" ("Enum"), error in (no error)=w174) -> (queue out=w176:refnum<queue>, error out=w173:errorcluster)  [unwired: 1 in, 1 out]
      }
    }
  }
  n49 = while {
    tunnel: w46 -> [w187]
    tunnel: w45 -> [w184]
    stop <- w181 stop-if-true
    # "Status Loop for Action Queues"
    n50 = Get Queue Status(queue=w187, return elements? (F)=TRUE) -> (error out=w183:errorcluster, # elements in queue=→"Action Queue Items":i32, elements=→"Action Queues items":string[])  [unwired: 1 in, 5 out]
    n51 = Get Queue Status(queue=w184, return elements? (F)=TRUE) -> (# pending remove=→"State Logic Queue Items":i32, error out=w182:errorcluster, elements=→"elements":T6[])  [unwired: 1 in, 5 out]
    n52 = Merge Errors(w183, w182) -> (w181:errorcluster)
    n53 = Wait (ms)(milliseconds to wait=u32 500) -> ()  [unwired: 1 out]
  }
  n54 = call "IMAQ Create"("Image Name"="Image dest") -> ("New Image"=w17:T19, "error out"=w16:errorcluster)  [unwired: 4 in]
  n55 = while {
    tunnel: w45 -> [w215]
    tunnel: w46 -> [w227]
    tunnel: w49 -> [w225]
    tunnel: [w224] -> _
    tunnel: [w223] -> w39
    shift-right: [w216] -> _
    shift-left: T11 {"PING_A"=0, "PING_B"=0, "PING_C"=0, "PING_D"=0} -> [w218]
    shift-right: [w209] -> _
    shift-left: State_Type_Definitions."Startup" ("Enum") -> [w212]
    shift-right: [w205] -> _
    shift-left: T12 {"xDistance"=0.0, "yDistance"=0.0, "wDistance"=0.0} -> [w207]
    shift-right: [w202] -> _
    shift-left: _ -> [w201]
    tunnel: w17 -> [w200]
    tunnel: w16 -> [w199]
    shift-right: [w196] -> _
    shift-left: T10 {"Recognized Object"=FALSE, "Object X coordinate"=0.0, "Object Y coordinate"=0.0} -> [w198]
    shift-right: [w193] -> _
    shift-left: T8 {"y Stepper Position"=0, "z Stepper Position"=0} -> [w195]
    shift-right: [w190] -> _
    shift-left: T7 {"Yaw"=0.0, "Compass"=0.0} -> [w192]
    stop <- w214 stop-if-true
    # ">>Error  >>"
    # ">>Action Queue>>"
    # ">>Timeout>>"
    # ">>Action states Queue Reference >>"
    # ">>State Logic Queue Reference >>"
    # "TOP LEVEL BASELINE (MAIN PROCESSING LOOP)"
    n56 = Dequeue Element(queue=w227, timeout in ms (-1)=0, error in (no error)=w225) -> (queue out=w219:refnum<queue>, element=w226:string, error out=w220:errorcluster)  [unwired: 1 out]
    "Action State" <- w226
    n57 = Wait (ms)(milliseconds to wait=u32 50) -> ()  [unwired: 1 out]
    n58 = case shown="\"RIGHT\"" w226 {
      tunnel: [_ _ _ _ _ _ _ _ _ _ _ _ _ _ _ _ 0 w863 _ _ _ _ _ _ _ _ _ _ _ _ _ _ _] -> w222
      tunnel: w219 -> [_ _ _ _ _ _ _ _ _ _ _ _ _ _ _ _ _ _ _ _ _ _ _ _ _ _ _ _ _ _ _ _ _]
      tunnel: w218 -> [w701 w708 w717 w726 w735 w744 w753 w762 w771 w776 w789 w801 w810 w817 w839 w847 w856 w864 w871 w878 w903 w912 w918 w925 w936 w947 w965 w975 w980 w988 w996 w1004 w1015]
      tunnel: [w701 w708 w717 w726 w735 w744 w753 w762 w771 w776 w789 w802 w810 w817 w840 w847 w856 w864 w871 w878 w902 w912 w918 w925 w936 w947 w965 w975 w980 w988 w996 w1004 w1015] -> w217
      tunnel: [TRUE TRUE _ _ _ _ _ _ _ _ _ _ _ _ _ _ _ _ _ _ _ _ _ _ _ _ _ _ _ _ _ _ _] -> w214
      tunnel: w212 -> [w699 w706 w716 w725 w734 w743 w752 w761 w770 w775 w788 w800 w809 w816 w838 w846 w853 w861 w870 w877 w901 w911 w917 w924 w930 w941 w964 w970 w979 w987 w995 w1003 w1014]
      tunnel: [_ _ _ _ _ _ _ _ _ _ _ _ _ _ _ _ _ TRUE _ _ _ _ _ _ _ _ _ _ _ _ _ _ _] -> w211
      tunnel: [w699 w706 w716 w725 w734 w743 w752 w761 w770 w775 w788 w800 w809 w816 w838 w846 w853 w861 w870 w877 w901 w911 w917 w924 w930 w941 w964 w970 w979 w987 w995 w1003 w1014] -> w210
      tunnel: w207 -> [w698 w705 w715 w724 w733 w742 w751 w760 w769 w777 w787 w799 w811 w818 w837 w848 w852 w860 w872 w879 w891 w910 w920 w926 w937 w948 w966 w976 w982 w990 w998 w1006 w1017]
      tunnel: [w698 w705 w715 w724 w733 w742 w751 w760 w769 w777 w786 w799 w811 w818 w836 w848 w852 w860 w872 w879 w890 w910 w920 w926 w937 w948 w966 w976 w982 w990 w998 w1006 w1017] -> w206
      tunnel: w200 -> [_ _ _ _ _ _ _ _ _ _ _ _ _ _ _ _ _ _ _ _ _ _ _ _ _ _ w959 _ _ _ _ _ _]
      tunnel: w199 -> [_ _ _ _ _ _ _ _ _ _ _ _ _ _ _ _ _ _ _ _ _ _ _ _ _ _ w958 _ _ _ _ _ _]
      tunnel: w198 -> [w697 w704 w714 w723 w732 w741 w749 w759 w768 w774 w785 w798 w803 w815 w828 w845 w851 w859 w869 w876 w896 w908 w919 w923 w929 w940 w957 w969 w981 w989 w997 w1005 w1016]
      tunnel: [w697 w704 w714 w723 w732 w741 w749 w759 w768 w774 w785 w798 w803 w815 w827 w845 w851 w859 w869 w876 w895 w908 w919 w923 w929 w940 w951 w969 w981 w989 w997 w1005 w1016] -> w197
      tunnel: w195 -> [w696 w703 w713 w722 w731 w740 w748 w758 w767 w773 w784 w797 w812 w814 w833 w844 w850 w858 w868 w875 w886 w907 w916 w922 w928 w939 w950 w968 w978 w986 w994 w1002 w1013]
      tunnel: [w696 w703 w713 w722 w731 w740 w748 w758 w767 w773 w784 w797 w812 w814 w832 w844 w850 w858 w868 w875 w885 w907 w916 w922 w928 w939 w950 w968 w978 w986 w994 w1002 w1012] -> w194
      tunnel: w192 -> [w695 w702 w712 w721 w730 w739 w747 w757 w766 w772 w778 w790 w807 w813 w823 w843 w849 w857 w867 w874 w882 w906 w913 w921 w927 w938 w949 w967 w977 w983 w991 w999 w1007]
      tunnel: [w695 w702 w712 w721 w730 w739 w747 w757 w766 w772 w778 w790 w806 w813 w822 w843 w849 w857 w867 w874 w881 w906 w913 w921 w927 w938 w949 w967 w977 w983 w991 w999 w1007] -> w191
      frame "Exit" {
        n59 = call "Imaq Dispose"("All Images? (No)"=TRUE) -> ()  [unwired: 5 in, 1 out]
      }
      frame "----Movement States----" {
      }
      frame "FORWARD" {
        n60 = call "Motor Control NO PID AE Ver.vi"("Direction"=MOTOR_CONTROL_NO_PID_AE_DIRECTIONS_type_def."y-axis movement", "AE Mode"=MOTOR_CONTROL_NO_PID_AE_DATA_ENTRY_MODE_Type_def."Write to motors", "Speed"=0.8) -> ()  [unwired: 2 in, 2 out]
      }
      frame "LEFT" {
        n61 = call "Motor Control NO PID AE Ver.vi"("Direction"=MOTOR_CONTROL_NO_PID_AE_DIRECTIONS_type_def."x-axis movement", "AE Mode"=MOTOR_CONTROL_NO_PID_AE_DATA_ENTRY_MODE_Type_def."Write to motors", "Speed"=-0.8) -> ()  [unwired: 2 in, 2 out]
      }
      frame "R-ACW" {
        n62 = call "Motor Control NO PID AE Ver.vi"("Direction"=MOTOR_CONTROL_NO_PID_AE_DIRECTIONS_type_def."Rotate", "AE Mode"=MOTOR_CONTROL_NO_PID_AE_DATA_ENTRY_MODE_Type_def."Write to motors", "Speed"=0.5) -> ()  [unwired: 2 in, 2 out]
      }
      frame "R-CW" {
        (unwired) -0.2 ("Speed")
        n63 = call "Motor Control NO PID AE Ver.vi"("Direction"=MOTOR_CONTROL_NO_PID_AE_DIRECTIONS_type_def."Rotate", "AE Mode"=MOTOR_CONTROL_NO_PID_AE_DATA_ENTRY_MODE_Type_def."Write to motors", "Speed"=-0.5) -> ()  [unwired: 2 in, 2 out]
      }
      frame "STOP" {
        n64 = Wait (ms)(milliseconds to wait=u32 200) -> ()  [unwired: 1 out]
        n65 = call "Motor Control NO PID AE Ver.vi"("Direction"=MOTOR_CONTROL_NO_PID_AE_DIRECTIONS_type_def."Stop", "AE Mode"=MOTOR_CONTROL_NO_PID_AE_DATA_ENTRY_MODE_Type_def."Write to motors") -> ()  [unwired: 3 in, 2 out]
      }
      frame "RIGHT" {
        n66 = call "Motor Control NO PID AE Ver.vi"("Direction"=MOTOR_CONTROL_NO_PID_AE_DIRECTIONS_type_def."x-axis movement", "AE Mode"=MOTOR_CONTROL_NO_PID_AE_DATA_ENTRY_MODE_Type_def."Write to motors", "Speed"=-0.8) -> ()  [unwired: 2 in, 2 out]
      }
      frame "REVERSE" {
        n67 = call "Motor Control NO PID AE Ver.vi"("Direction"=MOTOR_CONTROL_NO_PID_AE_DIRECTIONS_type_def."y-axis movement", "AE Mode"=MOTOR_CONTROL_NO_PID_AE_DATA_ENTRY_MODE_Type_def."Write to motors", "Speed"=-0.5) -> ()  [unwired: 2 in, 2 out]
      }
      frame "----SENSOR READING---- " {
      }
      frame "READ ENCODERS" {
        # ">>> Current encoder distance >>>"
        # ">>> Ultrasonic Sensors Detect >>>"
        n68 = call "Motor Control NO PID AE Ver.vi"("AE Mode"=MOTOR_CONTROL_NO_PID_AE_DATA_ENTRY_MODE_Type_def."Read from Encoders") -> ("Speed & distance"=w782:T27)  [unwired: 4 in, 1 out]
        n69 = Unbundle By Name(w782) -> ("xDistance"=w781:dbl, "yDistance"=w780:dbl, "wDistance"=w779:dbl)
        n70 = Bundle By Name(cluster=w787, "xDistance"=w781, "yDistance"=w780, "wDistance"=w779) -> (w786:T12)
      }
      frame "READ ULTRASONIC" {
        (unwired) navX_type_def."Read Values" ("Mode")
        (unwired) MOTOR_CONTROL_NO_PID_Type_Def."Latch" ("Direction")
        # ">>> Ultrasonic Sensors Detect >>>"
        # ">>> Object detection >>>"
        # ">>> Encoders >>>"
        # ">>> Stepper position >>>"
        # ">>> Yaw >>>"
        n71 = call "Arduino Interfacing VI.vi"("AE Mode"=Arduino_Interfacing."Read From Arduino") -> ("Arduino Data"=w795:T3)  [unwired: 3 in, 1 out]
        n72 = Unbundle By Name(w795) -> ("PING A"=w794:u8, "PING B"=w793:u8, "PING C"=w792:u8, "PING D"=w791:u8)
        n73 = Bundle By Name(cluster=w801, "PING_A"=w794, "PING_B"=w793, "PING_C"=w792, "PING_D"=w791) -> (w802:T11)
      }
      frame " READ YAW" {
        # ">>> Yaw >>>"
        # ">>> Ultrasonic Sensors Detect >>>"
        # ">>> Object detection >>>"
        # ">>> Encoders >>>"
        # ">>> Stepper position >>>"
        n74 = call "navX reading VI.vi"("Mode"=navX_type_def."Read Values") -> ("NavX Readings"=w805:T2)  [unwired: 2 in, 3 out]
        n75 = Unbundle By Name(w805) -> ("Yaw"=w804:dbl)
        n76 = Bundle By Name(cluster=w807, "Yaw"=w804) -> (w806:T7)
      }
      frame "----SYSTEM MODES----" {
        (unwired) I2C_MASTER_Type_Def."Last State" ("Arduino Mode")
        # ">>> Object detection >>>"
        # ">>> Yaw >>>"
        # ">>> Ultrasonic Sensors Detect >>>"
        # ">>> Encoders >>>"
        # ">>> Stepper position >>>"
      }
      frame "INIT" {
        w834 = u8 0
        w835 = 0.0
        # ">>> Object detection >>>"
        # ">>> Yaw >>>"
        # ">>> Ultrasonic Sensors Detect >>>"
        # ">>> Encoders >>>"
        # ">>> Stepper position >>>"
        # ">>State Logic  >>"
        n77 = call "Arduino Interfacing VI.vi"("AE Mode"=Arduino_Interfacing."Initialize") -> ()  [unwired: 3 in, 2 out]
        n78 = call "FGV Bool.vi"("Init/Read/Write State"=States_for_Action_Engine."Initialize") -> ()  [unwired: 2 in, 2 out]
        n79 = call "Motor Control NO PID AE Ver.vi"("AE Mode"=MOTOR_CONTROL_NO_PID_AE_DATA_ENTRY_MODE_Type_def."Initialize") -> ()  [unwired: 4 in, 2 out]
        n80 = Bundle By Name(cluster=w828, "Recognized Object"=FALSE, "Object X coordinate"=0.0, "Object Y coordinate"=0.0) -> (w827:T10)
        n81 = Bundle By Name(cluster=w833, "y Stepper Position"=u8 0, "z Stepper Position"=u8 0) -> (w832:T8)
        n82 = Bundle By Name(cluster=w837, "xDistance"=w835, "yDistance"=w835, "wDistance"=w835) -> (w836:T12)
        n83 = Bundle By Name(cluster=w839, "PING_A"=w834, "PING_B"=w834, "PING_C"=w834, "PING_D"=w834) -> (w840:T11)
        n84 = Bundle By Name(cluster=w823, "Yaw"=0.0) -> (w822:T7)
      }
      frame "ARDUINO - ULTRASONIC" {
        # ">>> Object detection >>>"
        # ">>> Yaw >>>"
        # ">>> Ultrasonic Sensors Detect >>>"
        # ">>> Encoders >>>"
        # ">>> Stepper position >>>"
        # ">>State Logic  >>"
        n85 = call "Arduino Interfacing VI.vi"("Data to Write"=I2C_MASTER_WRITE_NEW_Type_Def."Ultrasonic sensors", "AE Mode"=Arduino_Interfacing."Write to Arduino") -> ()  [unwired: 2 in, 2 out]
      }
      frame "NAVX CALIBRATE" {
        # ">>> Object detection >>>"
        # ">>> Yaw >>>"
        # ">>> Ultrasonic Sensors Detect >>>"
        # ">>> Encoders >>>"
        # ">>> Stepper position >>>"
        # ">>State Logic  >>"
        # "Adds a 15 second delay to the startup process \nfor the NavX to calibrate"
        n86 = Wait (ms)(milliseconds to wait=u32 5000) -> ()  [unwired: 1 out]
      }
      frame "NO ACTION", Default {
        (unwired) u8 0 ("y Stepper value")
        (unwired) TRUE ("Latch")
        (unwired) navX_type_def."Read Values" ("Mode")
        (unwired) MOTOR_CONTROL_NO_PID_Type_Def."Latch" ("Direction")
        # ">>> Object detection >>>"
        # ">>> Yaw >>>"
        # ">>> Ultrasonic Sensors Detect >>>"
        # ">>> Encoders >>>"
        # ">>> Stepper position >>>"
        # ">>State Logic  >>"
        n87 = case shown="4" w861 {
          tunnel: [0 100] -> w863
          frame 1, Default {
          }
          frame 4 {
          }
        }
      }
      frame "----RESET CASES----" {
        (unwired) I2C_MASTER_Type_Def."Last State" ("Arduino Mode")
        # ">>> Object detection >>>"
        # ">>> Yaw >>>"
        # ">>> Ultrasonic Sensors Detect >>>"
        # ">>> Encoders >>>"
        # ">>> Stepper position >>>"
        # ">>State Logic  >>"
      }
      frame "RESET ENCODERS" {
        # ">>> Object detection >>>"
        # ">>> Yaw >>>"
        # ">>> Ultrasonic Sensors Detect >>>"
        # ">>> Encoders >>>"
        # ">>> Stepper position >>>"
        # ">>State Logic  >>"
        n88 = call "Motor Control NO PID AE Ver.vi"("AE Mode"=MOTOR_CONTROL_NO_PID_AE_DATA_ENTRY_MODE_Type_def."Reset Encoders") -> ()  [unwired: 4 in, 2 out]
      }
      frame "RESET FLAGS" {
        (unwired) I2C_MASTER_Type_Def."Last State" ("Arduino Mode")
        # "Resets any software variables\nand/or non-critical states"
        n89 = Wait (ms)(milliseconds to wait=u32 20) -> ()  [unwired: 1 out]
        n90 = Bundle By Name(cluster=w896, "Recognized Object"=FALSE, "Object X coordinate"=0.0, "Object Y coordinate"=0.0) -> (w895:T10)
        n91 = Bundle By Name(cluster=w886, "y Stepper Position"=u8 0, "z Stepper Position"=u8 0) -> (w885:T8)
        n92 = Bundle By Name(cluster=w891, "xDistance"=0.0, "yDistance"=0.0, "wDistance"=0.0) -> (w890:T12)
        n93 = Bundle By Name(cluster=w903, "PING_A"=u8 0, "PING_B"=u8 0, "PING_C"=u8 0, "PING_D"=u8 0) -> (w902:T11)
        n94 = Bundle By Name(cluster=w882, "Yaw"=0.0) -> (w881:T7)
      }
      frame "RESET YAW" {
        n95 = Wait (ms)(milliseconds to wait=u32 100) -> ()  [unwired: 1 out]
        n96 = call "navX reading VI.vi"("Mode"=navX_type_def."Zero Yaw") -> ()  [unwired: 2 in, 4 out]
      }
      frame "RESET ARM" {
        n97 = call "Arduino Interfacing VI.vi"("Data to Write"=I2C_MASTER_WRITE_NEW_Type_Def."Soft Reset", "AE Mode"=Arduino_Interfacing."Write to Arduino") -> ()  [unwired: 2 in, 2 out]
      }
      frame "--------CAM STATES-------" {
      }
      frame "OPEN LOG CAM" {
        n98 = call "Low-Level Grab.vi"("States"=State_control."Initialise", "Session In"=T26 "cam0") -> ("error out"=w932:errorcluster, "Session Out"=w933:T26)  [unwired: 7 in, 1 out]
        n99 = call "Low-Level Grab.vi"("error in (no error)"=w932, "States"=State_control."Start camera", "Session In"=w933) -> ()  [unwired: 6 in, 3 out]
      }
      frame "OPEN LIFE CAM" {
        (unwired) MOTOR_CONTROL_NO_PID_Type_Def."Latch" ("Direction")
        (unwired) navX_type_def."Read Values" ("Mode")
        n100 = call "Low-Level Grab.vi"("States"=State_control."Initialise", "Session In"=T26 "cam1") -> ("error out"=w943:errorcluster, "Session Out"=w944:T26)  [unwired: 7 in, 1 out]
        n101 = call "Low-Level Grab.vi"("error in (no error)"=w943, "States"=State_control."Start camera", "Session In"=w944) -> ()  [unwired: 6 in, 3 out]
      }
      frame "CAM ACQ" {
        # ">>> Yaw >>>"
        # ">>> Stepper position >>>"
        # ">>> Encoders >>>"
        # ">>> Object detection >>>"
        # ">>> Ultrasonic Sensors Detect >>>"
        # "Object detection"
        n102 = call "Low-Level Grab.vi"("error in (no error)"=w958, "States"=State_control."Continuous Acquisition ") -> ("error out"=w961:errorcluster, "Image Out"=w962:T19)  [unwired: 7 in, 1 out]
        n103 = call "Object Detection SubVI.vi"("Error In"=w961, "Mode"="Object recognition mode", "Image Dest"=w959, "Image in"=w962) -> ("Object Center Coordinates"=w956:cluster{"x":sgl, "y":sgl}, "Object detection cluster"=w953:T1)  [unwired: 2 out]
        "Object detection cluster" <- w953
        "Object Center Coordinates" <- w956
        n104 = Unbundle By Name(w953) -> ("Object detected?"=w952:bool)
        n105 = Unbundle By Name(w956) -> ("x"=w955:sgl, "y"=w954:sgl)
        n106 = Bundle By Name(cluster=w957, "Recognized Object"=w952, "Object X coordinate"=w955, "Object Y coordinate"=w954) -> (w951:T10)
      }
      frame "CAM CLOSE" {
        (unwired) MOTOR_CONTROL_NO_PID_Type_Def."Latch" ("Direction")
        (unwired) navX_type_def."Read Values" ("Mode")
        n107 = call "Low-Level Grab.vi"("States"=State_control."Stop camera") -> ("error out"=w972:errorcluster, "Session Out"=w973:T26)  [unwired: 8 in, 1 out]
        n108 = call "Low-Level Grab.vi"("error in (no error)"=w972, "States"=State_control."Dispose all", "Session In"=w973) -> ()  [unwired: 6 in, 3 out]
      }
      frame "-----ARM ACTIONS-----" {
      }
      frame "CLOSE CLAW" {
        n109 = call "Arduino Interfacing VI.vi"("Data to Write"=I2C_MASTER_WRITE_NEW_Type_Def."Close Claw", "AE Mode"=Arduino_Interfacing."Write to Arduino") -> ()  [unwired: 2 in, 2 out]
      }
      frame "OPEN CLAW" {
        n110 = call "Arduino Interfacing VI.vi"("Data to Write"=I2C_MASTER_WRITE_NEW_Type_Def."Open Claw", "AE Mode"=Arduino_Interfacing."Write to Arduino") -> ()  [unwired: 2 in, 2 out]
      }
      frame "Z STEPPER CAM HEIGHT " {
        n111 = call "Arduino Interfacing VI.vi"("Data to Write"=I2C_MASTER_WRITE_NEW_Type_Def."zStepper 10k", "AE Mode"=Arduino_Interfacing."Write to Arduino") -> ()  [unwired: 2 in, 2 out]
      }
      frame "READ STEPPER VALUES" {
        n112 = call "Arduino Interfacing VI.vi"("AE Mode"=Arduino_Interfacing."Read From Arduino") -> ("Arduino Data"=w1010:T3)  [unwired: 3 in, 1 out]
        n113 = Unbundle By Name(w1010) -> ("y Stepper Position"=w1009:u8, "z Stepper Position"=w1008:u8)
        n114 = Bundle By Name(cluster=w1013, "y Stepper Position"=w1009, "z Stepper Position"=w1008) -> (w1012:T8)
      }
    }
    "State Logic" <- w210
    n115 = local read "TASK ENABLE"() -> (w204:bool)
    n116 = Not(x=w204) -> (.not. x?=w203:bool)
    n117 = case shown="True" w211 {
      tunnel: w215 -> [w236 w261]
      tunnel: w219 -> [w232 w263]
      tunnel: [w236 w261] -> w224
      tunnel: [w232 w264] -> w223
      tunnel: w220 -> [_ w259]
      tunnel: w222 -> [_ w260]
      tunnel: w217 -> [w235 w266]
      tunnel: [w235 w266] -> w216
      tunnel: "STOP TASK" -> [_ w249]
      tunnel: w210 -> [w234 w265]
      tunnel: [w234 w262] -> w209
      tunnel: w206 -> [w233 w255]
      tunnel: [w233 w255] -> w205
      tunnel: w203 -> [_ w250]
      tunnel: [w231 w247] -> w202
      tunnel: w201 -> [w231 w246]
      tunnel: w197 -> [w230 w243]
      tunnel: [w230 w243] -> w196
      tunnel: w194 -> [w229 w239]
      tunnel: [w229 w239] -> w193
      tunnel: w191 -> [w228 w237]
      tunnel: [w228 w237] -> w190
      frame False {
      }
      frame True {
        # ">>Action Queue>>"
        # ">>State Logic Queue Reference >>"
        n118 = Or(x=w249, y=w250) -> (x .or. y?=w248:bool)
        n119 = Unbundle By Name(w239) -> ("y Stepper Position"=w241:u8, "z Stepper Position"=w240:u8)
        n120 = Unbundle By Name(w255) -> ("xDistance"=w252:dbl, "yDistance"=w253:dbl, "wDistance"=w254:dbl)
        n121 = Unbundle By Name(w243) -> ("Recognized Object"=w242:bool, "Object X coordinate"=w245:dbl, "Object Y coordinate"=w244:dbl)
        n122 = Unbundle By Name(w266) -> ("PING_A"=w258:u8, "PING_B"=w257:u8, "PING_C"=w256:u8, "PING_D"=w251:u8)
        n123 = Unbundle By Name(w237) -> ("Yaw"=w238:dbl)
        n124 = case shown="7" w265 {
          tunnel: [w268 w271 w282 w289 w341 w353 w389 w435 w479 w536 w573 w625 w666] -> w264
          tunnel: w263 -> [w268 w274 w283 w292 w343 w354 w390 w436 w485 w529 w577 w620 w657]
          tunnel: [State_Type_Definitions."Idle" ("Enum") State_Type_Definitions."Idle" ("Enum") w278 w291 State_Type_Definitions."Shutdown" ("Enum") w355 w392 w434 w480 w535 w574 w626 w658] -> w262
          tunnel: w261 -> [_ _ w281 w295 _ w360 w402 w443 w484 w533 w578 w623 w665]
          tunnel: w260 -> [_ _ _ w294 _ w359 w401 w442 w483 w532 w570 w622 w663]
          tunnel: w259 -> [_ _ w280 w290 _ w358 w400 w441 w482 w531 w569 w621 w664]
          tunnel: w248 -> [_ _ _ _ _ w352 w391 w438 w478 w534 w575 w624 w661]
          tunnel: w258 -> [_ _ _ _ _ _ _ _ _ _ _ _ _]
          tunnel: w257 -> [_ _ _ _ _ _ w398 _ w476 w524 w580 _ _]
          tunnel: w256 -> [_ _ _ _ _ _ w397 _ w477 w525 w579 _ _]
          tunnel: w254 -> [_ _ _ _ _ _ _ w440 _ _ _ _ _]
          tunnel: w253 -> [_ _ _ _ _ w351 _ _ _ _ _ _ _]
          tunnel: w252 -> [_ _ _ _ _ _ _ _ _ w520 _ _ _]
          tunnel: w251 -> [_ _ _ _ _ _ _ _ _ _ _ _ _]
          tunnel: [State_Type_Definitions."Idle" ("Enum") State_Type_Definitions."Idle" ("Enum") State_Type_Definitions."Idle" ("Enum") State_Type_Definitions."Idle" ("Enum") State_Type_Definitions."Shutdown" ("Enum") w348 w388 w431 w471 w519 w572 w627 w659] -> w247
          tunnel: w246 -> [_ _ w278 _ _ _ _ _ _ _ _ _ _]
          tunnel: w242 -> [_ _ _ _ _ _ _ _ _ _ _ _ w660]
          tunnel: w245 -> [_ _ _ _ _ _ _ _ _ _ _ _ _]
          tunnel: w244 -> [_ _ _ _ _ _ _ _ _ _ _ _ _]
          tunnel: w241 -> [_ _ _ _ _ _ _ _ _ _ _ _ _]
          tunnel: w240 -> [_ _ _ _ _ _ _ _ _ _ _ w619 _]
          tunnel: w238 -> [_ _ _ _ _ _ _ _ _ _ _ _ _]
          frame 0 {
          }
          frame 1 {
            n125 = for {
              shift-right: [w277] -> w271
              shift-left: w274 -> [w276]
              tunnel: string[] ["INIT", "RESET ARM", "RESET FLAGS", "RESET YAW", "NAVX CALIBRATE"] -> [w275] mode=indexing
              n126 = Enqueue Element(queue=w276, element=w275) -> (queue out=w277:refnum<queue>)  [unwired: 2 in, 2 out]
            }
          }
          frame 3 {
            n127 = Flush Queue(queue=w281, error in (no error)=w280) -> ()  [unwired: 3 out]
            n128 = for {
              shift-right: [w287] -> w282
              shift-left: w283 -> [w286]
              tunnel: string[] ["STOP", "RESET ENCODERS", "RESET YAW", "ARDUINO MODE 0", "CAM CLOSE", "RESET ARM"] -> [w285] mode=indexing
              n129 = Enqueue Element(queue=w286, element=w285) -> (queue out=w287:refnum<queue>)  [unwired: 2 in, 2 out]
            }
          }
          frame 4, Default {
            (unwired) TRUE ("Green LED")
            n130 = Dequeue Element(queue=w295, timeout in ms (-1)=w294, error in (no error)=w290) -> (element=w293:T6)  [unwired: 3 out]
            n131 = case shown="\"Start Task 4\"" w293 {
              tunnel: [w297 w304 w311 w318 w325 w332 w334] -> w289
              tunnel: w292 -> [w298 w305 w312 w319 w326 w332 w335]
              tunnel: [State_Type_Definitions."Task 1" ("Enum") State_Type_Definitions."Task 2" ("Enum") State_Type_Definitions."Task 3" ("Enum") State_Type_Definitions."Task 4_A" ("Enum") State_Type_Definitions."Task 6_A" ("Enum") State_Type_Definitions."Idle" ("Enum") State_Type_Definitions."Shutdown" ("Enum")] -> w291
              frame "Start Task 1" {
                n132 = for {
                  shift-right: [w302] -> w297
                  shift-left: w298 -> [w301]
                  tunnel: string[] ["RESET ENCODERS", "RESET YAW", "FORWARD", "READ ENCODERS"] -> [w300] mode=indexing
                  n133 = Enqueue Element(queue=w301, element=w300) -> (queue out=w302:refnum<queue>)  [unwired: 2 in, 2 out]
                }
              }
              frame "Start Task 2" {
                n134 = for {
                  shift-right: [w309] -> w304
                  shift-left: w305 -> [w308]
                  tunnel: string[] ["RESET ENCODERS", "RESET YAW", "READ ULTRASONIC", "ARDUINO - ULTRASONIC"] -> [w307] mode=indexing
                  n135 = Enqueue Element(queue=w308, element=w307) -> (queue out=w309:refnum<queue>)  [unwired: 2 in, 2 out]
                }
              }
              frame "Start Task 3" {
                n136 = for {
                  shift-right: [w316] -> w311
                  shift-left: w312 -> [w315]
                  tunnel: string[] ["RESET ENCODERS", "READ ENCODERS", "R-ACW"] -> [w314] mode=indexing
                  n137 = Enqueue Element(queue=w315, element=w314) -> (queue out=w316:refnum<queue>)  [unwired: 2 in, 2 out]
                }
              }
              frame "Start Task 4" {
                n138 = for {
                  shift-right: [w323] -> w318
                  shift-left: w319 -> [w322]
                  tunnel: string[] ["STOP", "RESET YAW", "RESET ENCODERS", "READ ULTRASONIC", "ARDUINO - ULTRASONIC", ""] -> [w321] mode=indexing
                  n139 = Enqueue Element(queue=w322, element=w321) -> (queue out=w323:refnum<queue>)  [unwired: 2 in, 2 out]
                }
              }
              frame "Start Task 6" {
                n140 = for {
                  shift-right: [w330] -> w325
                  shift-left: w326 -> [w329]
                  tunnel: string[] ["Z STEPPER CAM HEIGHT ", "READ STEPPER VALUES", "OPEN LOG CAM", "", "", ""] -> [w328] mode=indexing
                  n141 = Enqueue Element(queue=w329, element=w328) -> (queue out=w330:refnum<queue>)  [unwired: 2 in, 2 out]
                }
              }
              frame "None", Default {
              }
              frame "Exit" {
                n142 = for {
                  shift-right: [w339] -> w334
                  shift-left: w335 -> [w338]
                  tunnel: string[] ["STOP", "RESET ENCODERS", "RESET YAW", "EXIT"] -> [w337] mode=indexing
                  n143 = Enqueue Element(queue=w338, element=w337) -> (queue out=w339:refnum<queue>)  [unwired: 2 in, 2 out]
                }
              }
            }
          }
          frame 5 {
            n144 = for {
              shift-right: [w347] -> w341
              shift-left: w343 -> [w346]
              tunnel: string[] ["INIT", "RESET ENCODERS", "RESET FLAGS", "EXIT"] -> [w345] mode=indexing
              n145 = Enqueue Element(queue=w346, element=w345) -> (queue out=w347:refnum<queue>)  [unwired: 2 in, 2 out]
            }
          }
          frame 6 {
            # "Use 250"
            n146 = Dequeue Element(queue=w360, timeout in ms (-1)=w359, error in (no error)=w358) -> (element=w357:T6)  [unwired: 3 out]
            n147 = Greater?(x=w351, y=250.0) -> (0:w349:bool)
            n148 = Or(x=w349, y=w352) -> (x .or. y?=w356:bool)
            n149 = case shown="\"None\", Default" w357 {
              tunnel: w356 -> [w363 _]
              tunnel: [w367 State_Type_Definitions."True Stop" ("Enum")] -> w355
              tunnel: w354 -> [w364 w382]
              tunnel: [w362 w381] -> w353
              tunnel: [State_Type_Definitions."Idle" ("Enum") State_Type_Definitions."Shutdown" ("Enum")] -> w348
              frame "None", Default {
                n150 = case shown="True" w363 {
                  tunnel: w364 -> [w370 w376]
                  tunnel: [w369 w374] -> w362
                  frame False {
                    n151 = for {
                      shift-right: [w372] -> w369
                      shift-left: w370 -> [w373]
                      tunnel: string[] ["READ ENCODERS", "READ YAW", "FORWARD"] ("element") -> [w371] mode=indexing
                      n152 = Enqueue Element(queue=w373, element=w371) -> (queue out=w372:refnum<queue>)  [unwired: 2 in, 2 out]
                    }
                  }
                  frame True {
                    n153 = for {
                      shift-right: [w378] -> w374
                      shift-left: w376 -> [w379]
                      tunnel: string[] ["RESET YAW", "RESET ENCODERS", "STOP", ""] -> [w377] mode=indexing
                      n154 = Enqueue Element(queue=w379, element=w377) -> (queue out=w378:refnum<queue>)  [unwired: 2 in, 2 out]
                    }
                  }
                }
                n155 = Select(t=State_Type_Definitions."True Stop" ("Enum"), s=w363, f=State_Type_Definitions."Task 1" ("Enum")) -> (s? t:f=w367:u16)
              }
              frame "Exit" {
                n156 = for {
                  shift-right: [w386] -> w381
                  shift-left: w382 -> [w387]
                  tunnel: string[] ["STOP", "RESET ENCODERS", "RESET YAW", ""] -> [w385] mode=indexing
                  n157 = Enqueue Element(queue=w387, element=w385) -> (queue out=w386:refnum<queue>)  [unwired: 2 in, 2 out]
                }
              }
            }
          }
          frame 7 {
            w396 = u16 10 ("y")
            # ">>Object detected>>"
            n158 = Dequeue Element(queue=w402, timeout in ms (-1)=w401, error in (no error)=w400) -> (element=w399:T6)  [unwired: 3 out]
            n159 = Less?(x=w398, y=w396) -> (x < y?=w395:bool)
            n160 = Less?(x=w397, y=w396) -> (x < y?=w394:bool)
            n161 = Or(x=w395, y=w394) -> (x .or. y?=w393:bool)
            "Object detected?" <- w393
            n162 = case shown="\"None\", Default" w399 {
              tunnel: w393 -> [w406 _]
              tunnel: [w408 State_Type_Definitions."True Stop" ("Enum")] -> w392
              tunnel: w391 -> [w407 _]
              tunnel: w390 -> [w405 w425]
              tunnel: [w404 w426] -> w389
              tunnel: [State_Type_Definitions."Idle" ("Enum") State_Type_Definitions."Shutdown" ("Enum")] -> w388
              frame "None", Default {
                n163 = case shown="False" w406 {
                  tunnel: w405 -> [w412 w419]
                  tunnel: [w413 w418] -> w404
                  frame False {
                    n164 = for {
                      tunnel: string[] ["READ ULTRASONIC", "STOP"] ("element") -> [w414] mode=indexing
                      shift-right: [w416] -> w413
                      shift-left: w412 -> [w415]
                      n165 = Enqueue Element(queue=w415, element=w414) -> (queue out=w416:refnum<queue>)  [unwired: 2 in, 2 out]
                    }
                  }
                  frame True {
                    n166 = for {
                      shift-right: [w421] -> w418
                      shift-left: w419 -> [w422]
                      tunnel: string[] ["REVERSE", "READ ULTRASONIC"] -> [w420] mode=indexing
                      n167 = Enqueue Element(queue=w422, element=w420) -> (queue out=w421:refnum<queue>)  [unwired: 2 in, 2 out]
                    }
                  }
                }
                n168 = Select(t=State_Type_Definitions."True Stop" ("Enum"), s=w407, f=State_Type_Definitions."Task 2" ("Enum")) -> (s? t:f=w408:u16)
              }
              frame "Exit" {
                n169 = for {
                  shift-right: [w429] -> w426
                  shift-left: w425 -> [w430]
                  tunnel: string[] ["STOP", "RESET ENCODERS", "RESET YAW", "ARDUINO MODE 0"] -> [w428] mode=indexing
                  n170 = Enqueue Element(queue=w430, element=w428) -> (queue out=w429:refnum<queue>)  [unwired: 2 in, 2 out]
                }
              }
            }
          }
          frame 10 {
            n171 = Dequeue Element(queue=w443, timeout in ms (-1)=w442, error in (no error)=w441) -> (element=w432:T6)  [unwired: 3 out]
            n172 = Greater?(x=w440, y=150.0) -> (0:w437:bool)
            n173 = Or(x=w437, y=w438) -> (x .or. y?=w433:bool)
            n174 = case shown="\"Exit\"" w432 {
              tunnel: w433 -> [w446 _]
              tunnel: [w450 State_Type_Definitions."True Stop" ("Enum")] -> w434
              tunnel: w436 -> [w447 w466]
              tunnel: [w445 w465] -> w435
              tunnel: [State_Type_Definitions."Idle" ("Enum") State_Type_Definitions."Shutdown" ("Enum")] -> w431
              frame "None", Default {
                n175 = case shown="False" w446 {
                  tunnel: w447 -> [w453 w459]
                  tunnel: [w452 w457] -> w445
                  frame False {
                    n176 = for {
                      shift-right: [w455] -> w452
                      shift-left: w453 -> [w456]
                      tunnel: string[] ["READ ENCODERS", "R-ACW"] ("element") -> [w454] mode=indexing
                      n177 = Enqueue Element(queue=w456, element=w454) -> (queue out=w455:refnum<queue>)  [unwired: 2 in, 2 out]
                    }
                  }
                  frame True {
                    n178 = for {
                      shift-right: [w461] -> w457
                      shift-left: w459 -> [w462]
                      tunnel: string[] ["RESET YAW", "RESET ENCODERS", "STOP", "ARDUINO MODE 0"] -> [w460] mode=indexing
                      n179 = Enqueue Element(queue=w462, element=w460) -> (queue out=w461:refnum<queue>)  [unwired: 2 in, 2 out]
                    }
                  }
                }
                n180 = Select(t=State_Type_Definitions."True Stop" ("Enum"), s=w446, f=State_Type_Definitions."Task 3" ("Enum")) -> (s? t:f=w450:T5)
              }
              frame "Exit" {
                n181 = for {
                  shift-right: [w469] -> w465
                  shift-left: w466 -> [w470]
                  tunnel: string[] ["STOP", "RESET ENCODERS", "RESET YAW", ""] -> [w468] mode=indexing
                  n182 = Enqueue Element(queue=w470, element=w468) -> (queue out=w469:refnum<queue>)  [unwired: 2 in, 2 out]
                }
              }
            }
          }
          frame 11 {
            w475 = 20
            # ">> Outputs true if object detected >>"
            # ">> Manual override >>"
            n183 = Dequeue Element(queue=w484, timeout in ms (-1)=w483, error in (no error)=w482) -> (element=w481:T6)  [unwired: 3 out]
            n184 = Less?(x=w477, y=w475) -> (x < y?=w473:bool)
            n185 = Less?(x=w476, y=w475) -> (x < y?=w474:bool)
            n186 = And(x=w474, y=w473) -> (x .and. y?=w472:bool)
            "Detect?" <- w472
            n187 = case shown="\"None\", Default" w481 {
              tunnel: [w494 State_Type_Definitions."True Stop" ("Enum")] -> w480
              tunnel: [w492 w513] -> w479
              tunnel: w485 -> [w491 _]
              tunnel: w478 -> [w489 _]
              tunnel: w472 -> [w487 _]
              tunnel: [w486 State_Type_Definitions."Shutdown" ("Enum")] -> w471
              frame "None", Default {
                # ">> WIill proceed to part ii if not manual override >>"
                # ">>If ENABLE or Trigger is set to true>>"
                n188 = Or(x=w487, y=w489) -> (x .or. y?=w488:bool)
                n189 = case shown="False" w488 {
                  tunnel: [w501 w506] -> w492
                  tunnel: w491 -> [w499 w505]
                  frame False {
                    n190 = for {
                      shift-right: [w503] -> w501
                      shift-left: w499 -> [w504]
                      tunnel: string[] ["FORWARD", "ULTRASONIC READ", ""] ("element") -> [w502] mode=indexing
                      n191 = Enqueue Element(queue=w504, element=w502) -> (queue out=w503:refnum<queue>)  [unwired: 2 in, 2 out]
                    }
                  }
                  frame True {
                    n192 = for {
                      shift-right: [w509] -> w506
                      shift-left: w505 -> [w510]
                      tunnel: string[] ["STOP", "RESET ENCODERS", "RESET YAW", "ARDUINO MODE 0"] -> [w508] mode=indexing
                      n193 = Enqueue Element(queue=w510, element=w508) -> (queue out=w509:refnum<queue>)  [unwired: 2 in, 2 out]
                    }
                  }
                }
                n194 = case shown="False" w489 {
                  tunnel: [State_Type_Definitions."True Stop" ("Enum") State_Type_Definitions."True Stop" ("Enum")] -> w490
                  tunnel: [State_Type_Definitions."Task 4_B" ("Enum") State_Type_Definitions."Idle" ("Enum")] -> w486
                  frame False {
                  }
                  frame True {
                  }
                }
                n195 = Select(t=w490, s=w488, f=State_Type_Definitions."Task 4_A" ("Enum")) -> (s? t:f=w494:T5)
              }
              frame "Exit" {
                n196 = for {
                  shift-right: [w516] -> w513
                  shift-left: _ -> [w517]
                  tunnel: string[] ["STOP", "RESET ENCODERS", "RESET YAW", ""] -> [w515] mode=indexing
                  n197 = Enqueue Element(queue=w517, element=w515) -> (queue out=w516:refnum<queue>)  [unwired: 2 in, 2 out]
                }
              }
            }
          }
          frame 12 {
            w528 = 20
            # ">> Outputs true if 150 mm has been moved >>"
            # ">> Outputs true if sensor not obstructed>>"
            # ">> Manual override >>"
            n198 = Dequeue Element(queue=w533, timeout in ms (-1)=w532, error in (no error)=w531) -> (element=w530:T6)  [unwired: 3 out]
            n199 = Greater?(x=w525, y=w528) -> (0:w526:bool)
            n200 = Greater?(x=w524, y=w528) -> (0:w527:bool)
            n201 = Greater Or Equal?(x=w520, y=80.0) -> (x >= y?=w522:bool)
            n202 = And(x=w527, y=w526) -> (x .and. y?=w521:bool)
            n203 = And(x=w522, y=w521) -> (x .and. y?=w518:bool)
            n204 = case shown="\"None\", Default" w530 {
              tunnel: [w545 State_Type_Definitions."True Stop" ("Enum")] -> w535
              tunnel: [w543 w564] -> w536
              tunnel: w529 -> [w542 _]
              tunnel: w534 -> [w540 _]
              tunnel: w518 -> [w538 _]
              tunnel: [w537 State_Type_Definitions."Shutdown" ("Enum")] -> w519
              frame "None", Default {
                # ">> WIill proceed to part ii if not manual override >>"
                # ">>If ENABLE or Trigger is set to true>>"
                n205 = Or(x=w538, y=w540) -> (x .or. y?=w539:bool)
                n206 = case shown="False" w539 {
                  tunnel: [w552 w557] -> w543
                  tunnel: w542 -> [w550 w556]
                  frame False {
                    n207 = for {
                      shift-right: [w554] -> w552
                      shift-left: w550 -> [w555]
                      tunnel: string[] ["RIGHT", "ULTRASONIC READ", "READ ENCODERS"] ("element") -> [w553] mode=indexing
                      n208 = Enqueue Element(queue=w555, element=w553) -> (queue out=w554:refnum<queue>)  [unwired: 2 in, 2 out]
                    }
                  }
                  frame True {
                    n209 = for {
                      shift-right: [w560] -> w557
                      shift-left: w556 -> [w561]
                      tunnel: string[] ["STOP", "RESET ENCODERS", "RESET YAW", "ARDUINO MODE 0"] -> [w559] mode=indexing
                      n210 = Enqueue Element(queue=w561, element=w559) -> (queue out=w560:refnum<queue>)  [unwired: 2 in, 2 out]
                    }
                  }
                }
                n211 = case shown="True" w540 {
                  tunnel: [State_Type_Definitions."True Stop" ("Enum") State_Type_Definitions."True Stop" ("Enum")] -> w541
                  tunnel: [State_Type_Definitions."Task 4_C" ("Enum") State_Type_Definitions."Idle" ("Enum")] -> w537
                  frame False {
                  }
                  frame True {
                  }
                }
                n212 = Select(t=w541, s=w539, f=State_Type_Definitions."Task 4_B" ("Enum")) -> (s? t:f=w545:T5)
              }
              frame "Exit" {
                n213 = for {
                  shift-right: [w567] -> w564
                  shift-left: _ -> [w568]
                  tunnel: string[] ["STOP", "RESET ENCODERS", "RESET YAW", ""] -> [w566] mode=indexing
                  n214 = Enqueue Element(queue=w568, element=w566) -> (queue out=w567:refnum<queue>)  [unwired: 2 in, 2 out]
                }
              }
            }
          }
          frame 13 {
            w583 = 20
            # ">> Outputs true if object detected >>"
            # ">> Manual override >>"
            n215 = Dequeue Element(queue=w578, timeout in ms (-1)=w570, error in (no error)=w569) -> (element=w571:T6)  [unwired: 3 out]
            n216 = Less?(x=w579, y=w583) -> (x < y?=w581:bool)
            n217 = Less?(x=w580, y=w583) -> (x < y?=w582:bool)
            n218 = And(x=w582, y=w581) -> (x .and. y?=w576:bool)
            n219 = case shown="\"None\", Default" w571 {
              tunnel: [w592 State_Type_Definitions."True Stop" ("Enum")] -> w574
              tunnel: [w590 w612] -> w573
              tunnel: w577 -> [w589 w609]
              tunnel: w575 -> [w587 _]
              tunnel: w576 -> [w585 _]
              tunnel: [w584 State_Type_Definitions."Shutdown" ("Enum")] -> w572
              frame "None", Default {
                # ">> WIill proceed to part ii if not manual override >>"
                # ">>If ENABLE or Trigger is set to true>>"
                n220 = Or(x=w585, y=w587) -> (x .or. y?=w586:bool)
                n221 = case shown="False" w586 {
                  tunnel: [w599 w604] -> w590
                  tunnel: w589 -> [w597 w603]
                  frame False {
                    n222 = for {
                      shift-right: [w601] -> w599
                      shift-left: w597 -> [w602]
                      tunnel: string[] ["FORWARD", "ULTRASONIC READ", ""] ("element") -> [w600] mode=indexing
                      n223 = Enqueue Element(queue=w602, element=w600) -> (queue out=w601:refnum<queue>)  [unwired: 2 in, 2 out]
                    }
                  }
                  frame True {
                    n224 = for {
                      shift-right: [w607] -> w604
                      shift-left: w603 -> [w608]
                      tunnel: string[] ["STOP", "RESET ENCODERS", "RESET YAW", "ARDUINO MODE 0"] -> [w606] mode=indexing
                      n225 = Enqueue Element(queue=w608, element=w606) -> (queue out=w607:refnum<queue>)  [unwired: 2 in, 2 out]
                    }
                  }
                }
                n226 = case shown="True" w587 {
                  tunnel: [State_Type_Definitions."True Stop" ("Enum") State_Type_Definitions."True Stop" ("Enum")] -> w588
                  tunnel: [State_Type_Definitions."Idle" ("Enum") State_Type_Definitions."Idle" ("Enum")] -> w584
                  frame False {
                  }
                  frame True {
                  }
                }
                n227 = Select(t=w588, s=w586, f=State_Type_Definitions."Task 4_C" ("Enum")) -> (s? t:f=w592:T5)
              }
              frame "Exit" {
                n228 = for {
                  shift-right: [w615] -> w612
                  shift-left: w609 -> [w616]
                  tunnel: string[] ["STOP", "RESET ENCODERS", "RESET YAW", ""] -> [w614] mode=indexing
                  n229 = Enqueue Element(queue=w616, element=w614) -> (queue out=w615:refnum<queue>)  [unwired: 2 in, 2 out]
                }
              }
            }
          }
          frame 23 {
            (unwired) u16 10 ("y")
            n230 = Dequeue Element(queue=w623, timeout in ms (-1)=w622, error in (no error)=w621) -> (element=w628:T6)  [unwired: 3 out]
            n231 = Equal?(x=w619, y=u8 100) -> (x = y?=w618:bool)
            n232 = case shown="\"None\", Default" w628 {
              tunnel: [w635 State_Type_Definitions."True Stop" ("Enum")] -> w626
              tunnel: [w634 w652] -> w625
              tunnel: [State_Type_Definitions."Idle" ("Enum") State_Type_Definitions."Shutdown" ("Enum")] -> w627
              tunnel: w624 -> [w630 _]
              tunnel: w620 -> [w632 _]
              tunnel: w618 -> [w629 _]
              frame "None", Default {
                n233 = case shown="False" w629 {
                  tunnel: [w640 w646] -> w634
                  tunnel: w632 -> [w638 w644]
                  frame False {
                    n234 = for {
                      tunnel: string[] ["Z STEPPER CAM HEIGHT", "READ STEPPER VALUES"] ("element") -> [w641] mode=indexing
                      shift-right: [w643] -> w640
                      shift-left: w638 -> [w642]
                      n235 = Enqueue Element(queue=w642, element=w641) -> (queue out=w643:refnum<queue>)  [unwired: 2 in, 2 out]
                    }
                  }
                  frame True {
                    n236 = for {
                      shift-right: [w648] -> w646
                      shift-left: w644 -> [w649]
                      tunnel: string[] ["CAM ACQ", ""] -> [w647] mode=indexing
                      n237 = Enqueue Element(queue=w649, element=w647) -> (queue out=w648:refnum<queue>)  [unwired: 2 in, 2 out]
                    }
                  }
                }
                n238 = Or(x=w629, y=w630) -> (x .or. y?=w631:bool)
                n239 = Select(t=State_Type_Definitions."Task 6_B" ("Enum"), s=w631, f=State_Type_Definitions."Task 6_A" ("Enum")) -> (s? t:f=w635:T5)
              }
              frame "Exit" {
                n240 = for {
                  shift-right: [w655] -> w652
                  shift-left: _ -> [w656]
                  tunnel: string[] ["STOP", "RESET ENCODERS", "RESET YAW", "ARDUINO MODE 0"] -> [w654] mode=indexing
                  n241 = Enqueue Element(queue=w656, element=w654) -> (queue out=w655:refnum<queue>)  [unwired: 2 in, 2 out]
                }
              }
            }
          }
          frame 24 {
            n242 = Dequeue Element(queue=w665, timeout in ms (-1)=w663, error in (no error)=w664) -> (element=w662:T6)  [unwired: 3 out]
            n243 = case shown="\"None\", Default" w662 {
              tunnel: [w672 State_Type_Definitions."True Stop" ("Enum")] -> w658
              tunnel: [w671 w689] -> w666
              tunnel: [State_Type_Definitions."Idle" ("Enum") State_Type_Definitions."Shutdown" ("Enum")] -> w659
              tunnel: w661 -> [w667 _]
              tunnel: w660 -> [w669 _]
              tunnel: w657 -> [w668 _]
              frame "None", Default {
                n244 = case shown="True" w669 {
                  tunnel: [w677 w683] -> w671
                  tunnel: w668 -> [w676 w681]
                  frame False {
                    n245 = for {
                      shift-right: [w680] -> w677
                      shift-left: w676 -> [w679]
                      tunnel: string[] ["CAM ACQ", "OPEN CLAW"] -> [w678] mode=indexing
                      n246 = Enqueue Element(queue=w679, element=w678) -> (queue out=w680:refnum<queue>)  [unwired: 2 in, 2 out]
                    }
                  }
                  frame True {
                    n247 = for {
                      shift-right: [w685] -> w683
                      shift-left: w681 -> [w686]
                      tunnel: string[] ["CAM ACQ", "CLOSE CLAW"] -> [w684] mode=indexing
                      n248 = Enqueue Element(queue=w686, element=w684) -> (queue out=w685:refnum<queue>)  [unwired: 2 in, 2 out]
                    }
                  }
                }
                n249 = Select(t=State_Type_Definitions."True Stop" ("Enum"), s=w667, f=State_Type_Definitions."Task 6_B" ("Enum")) -> (s? t:f=w672:T5)
              }
              frame "Exit" {
                n250 = for {
                  shift-right: [w692] -> w689
                  shift-left: _ -> [w693]
                  tunnel: string[] ["STOP", "RESET ENCODERS", "RESET YAW", "ARDUINO MODE 0"] -> [w691] mode=indexing
                  n251 = Enqueue Element(queue=w693, element=w691) -> (queue out=w692:refnum<queue>)  [unwired: 2 in, 2 out]
                }
              }
            }
          }
        }
      }
    }
  }
  n252 = call <vilib>:"DIO Close.vi"("error in (no error)"=w22, "DIO Info In"=w25) -> ()  [unwired: 9 in, 1 out]
  n253 = call <vilib>:"DIO Close.vi"("error in (no error)"=w32, "DIO Info In"=w34) -> ()  [unwired: 9 in, 1 out]
  n254 = call <vilib>:"NavX Close.vi"("error in (no error)"=w3, "NavX Info In"=w2) -> ()  [unwired: 9 in, 1 out]
  n255 = call <vilib>:"DIO Close.vi"("error in (no error)"=w27, "DIO Info In"=w29) -> ()  [unwired: 9 in, 1 out]
  n256 = call <vilib>:"DIO Close.vi"("error in (no error)"=w10, "DIO Info In"=w11) -> ()  [unwired: 9 in, 1 out]
  n257 = call <vilib>:"DIO Close.vi"("error in (no error)"=w5, "DIO Info In"=w6) -> ()  [unwired: 9 in, 1 out]
  n258 = while {
    stop <- w1019 stop-if-true
    n259 = call <vilib>:"RT Get CPU Loads.vi"() -> ("CPU loads"=→"CPU loads":T4[])  [unwired: 10 in, 1 out]
    n260 = Wait (ms)(milliseconds to wait=u32 100) -> ()  [unwired: 1 out]
    n261 = call "FGV Bool.vi"("Init/Read/Write State"=States_for_Action_Engine."Read") -> ("Output node"=w1019:bool)  [unwired: 2 in, 1 out]
  }
  n262 = Merge Errors "Merge Errors"(w62, w61) -> (w44:errorcluster)
  n263 = Merge Errors(w48, w44) -> (w43:errorcluster)
  n264 = Destroy User Event(user event=w65, error in=w43) -> ()  [unwired: 1 out]
  n265 = Destroy User Event(user event=w66, error in=w43) -> ()  [unwired: 1 out]
  n266 = Unregister For Events(event registration refnum=w57, error in=w43) -> ()  [unwired: 1 out]
  n267 = Release Queue(queue=w39, error in (no error)=w43) -> (error out=w21:errorcluster)  [unwired: 1 in, 2 out]
  n268 = Release Queue(queue=w56, error in (no error)=w43) -> ()  [unwired: 1 in, 3 out]
  n269 = call <vilib>:"Simple Error Handler.vi"("error in (no error)"=w21) -> ("error out"=w20:errorcluster)  [unwired: 4 in, 4 out]
  n270 = call <vilib>:"Reset myRIO.vi"("error in (no error)"=w20) -> ("error out"=→"error out":errorcluster)  [unwired: 10 in]
